vi "Customized NA.vi"() -> ()   [LabVIEW 2021]
panel:
  out "A 2":dbl
  out "A":dbl
  out "Transmission":cluster{"X":dbl, "Y":dbl}[](graph)=[{"X"=1.0, "Y"=0.022832684978800612}, {"X"=1.01, "Y"=-0.03508112044447924}, {"X"=1.02, "Y"=0.011268875649849798}, {"X"=1.03, "Y"=-0.0005874144163142788}, {"X"=1.04, "Y"=-0.013460551415189913}, {"X"=1.05, "Y"=-0.0028755295385605416}, {"X"=1.06, "Y"=-0.01981361181122932}, {"X"=1.07, "Y"=-0.01643174646657092}, {"X"=1.08, "Y"=-0.009902749417672363}, {"X"=1.09, "Y"=0.02696994725538056}, {"X"=1.1, "Y"=0.0013856868529792457}, {"X"=1.11, "Y"=-0.01094619808605209}, {"X"=1.12, "Y"=0.014859773774399874}, {"X"=1.13, "Y"=-0.027897423308499814}, {"X"=1.1400000000000001, "Y"=-0.027737684416107827}, {"X"=1.15, "Y"=0.007918297120363972}, {"X"=1.16, "Y"=-0.018397039322749057}, {"X"=1.17, "Y"=-0.014214660968136495}, {"X"=1.18, "Y"=0.05134840789052823}, {"X"=1.19, "Y"=0.006926672201586222}, {"X"=1.2, "Y"=0.020462736392556753}, {"X"=1.21, "Y"=-0.028066215237332482}, {"X"=1.22, "Y"=-0.02445743439576179}, {"X"=1.23, "Y"=0.03564938650047041}, {"X"=1.24, "Y"=-0.010377576540651738}, {"X"=1.25, "Y"=0.013453196897726083}, {"X"=1.26, "Y"=0.015431438626936772}, {"X"=1.27, "Y"=0.02283777498421219}, {"X"=1.28, "Y"=-0.007799579257767735}, {"X"=1.29, "Y"=0.0234923784994419}, {"X"=1.3, "Y"=0.020565792635922966}, {"X"=1.31, "Y"=0.014042606014675805}, {"X"=1.32, "Y"=-0.00826649286668001}, {"X"=1.33, "Y"=-0.007935280043591663}, {"X"=1.34, "Y"=0.03503153061398124}, {"X"=1.35, "Y"=0.026956957824188083}, {"X"=1.3599999999999999, "Y"=0.029441710251826573}, {"X"=1.37, "Y"=0.03176793153897496}, {"X"=1.38, "Y"=0.02707736760646512}, {"X"=1.3900000000000001, "Y"=0.002384192541336166}, {"X"=1.4, "Y"=-0.0042640262941606175}, {"X"=1.4100000000000001, "Y"=0.05346182081654834}, {"X"=1.42, "Y"=0.03555493439663364}, {"X"=1.43, "Y"=-0.004520863626681091}, {"X"=1.44, "Y"=-0.016774217224386375}, {"X"=1.45, "Y"=-0.005965400673648759}, {"X"=1.46, "Y"=-0.0010894043039113353}, {"X"=1.47, "Y"=-0.00046876709353084185}, {"X"=1.48, "Y"=0.012684810390652803}, {"X"=1.49, "Y"=0.03813067356398994}, {"X"=1.5, "Y"=0.028034897066981875}, {"X"=1.51, "Y"=0.0004972634699936428}, {"X"=1.52, "Y"=-0.00885702548596945}, {"X"=1.53, "Y"=-0.0014397783600446864}, {"X"=1.54, "Y"=0.02559738967135176}, {"X"=1.55, "Y"=0.02940201090770585}, {"X"=1.56, "Y"=-0.00800150373652454}, {"X"=1.57, "Y"=0.006450333329645636}, {"X"=1.58, "Y"=0.004569407290840438}, {"X"=1.5899999999999999, "Y"=-0.000598240579322772}, {"X"=1.6, "Y"=-0.014320673486041196}, {"X"=1.6099999999999999, "Y"=0.0027199883542179957}, {"X"=1.62, "Y"=0.02908043278181352}, {"X"=1.63, "Y"=0.020256081684782996}, {"X"=1.6400000000000001, "Y"=0.014829149563513153}, {"X"=1.65, "Y"=-0.019887629125237172}, {"X"=1.6600000000000001, "Y"=0.04144270630923306}, {"X"=1.67, "Y"=0.055620811367091655}, {"X"=1.6800000000000002, "Y"=-0.05015047761465842}, {"X"=1.69, "Y"=0.016115782004926103}, {"X"=1.7000000000000002, "Y"=0.022219967844359437}, {"X"=1.71, "Y"=-0.019533017885574717}, {"X"=1.72, "Y"=0.002002035002969814}, {"X"=1.73, "Y"=-0.018597470141180916}, {"X"=1.74, "Y"=-0.020507493473050777}, {"X"=1.75, "Y"=0.04497118743572116}, {"X"=1.76, "Y"=-0.03014262884386368}, {"X"=1.77, "Y"=-0.02635719806032388}, {"X"=1.78, "Y"=0.006535826712424916}, {"X"=1.79, "Y"=0.02334340013557594}, {"X"=1.8, "Y"=-0.014584642495372427}, {"X"=1.81, "Y"=0.030318500830231188}, {"X"=1.82, "Y"=0.020334854112019567}, {"X"=1.83, "Y"=0.04329884774917375}, {"X"=1.8399999999999999, "Y"=-0.025542094923208684}, {"X"=1.85, "Y"=0.003997116512462377}, {"X"=1.8599999999999999, "Y"=0.002476500606431811}, {"X"=1.87, "Y"=-0.015934904275146204}, {"X"=1.88, "Y"=0.022274962013573}, {"X"=1.8900000000000001, "Y"=-0.017679939353418044}, {"X"=1.9, "Y"=-0.006070507215851479}, {"X"=1.9100000000000001, "Y"=0.020445304004784615}, {"X"=1.92, "Y"=0.0240972950297685}, {"X"=1.9300000000000002, "Y"=-0.007427137567462293}, {"X"=1.94, "Y"=-0.04383462926305039}, {"X"=1.9500000000000002, "Y"=0.029534523383703232}, {"X"=1.96, "Y"=0.004663156332775081}, {"X"=1.97, "Y"=0.006710309156515723}, {"X"=1.98, "Y"=0.01918446886521864}, {"X"=1.99, "Y"=0.015197749143457322}, {"X"=2.0, "Y"=-0.009373297526692696}, {"X"=2.01, "Y"=-0.020787679571358297}, {"X"=2.02, "Y"=0.010482467499636692}, {"X"=2.0300000000000002, "Y"=-0.005673220895538561}, {"X"=2.04, "Y"=0.043413707084557746}, {"X"=2.05, "Y"=-0.035716121505957696}, {"X"=2.06, "Y"=0.009439154355609746}, {"X"=2.0700000000000003, "Y"=0.024819571500530446}, {"X"=2.08, "Y"=-0.016880198106777607}, {"X"=2.09, "Y"=0.026621278695482094}, {"X"=2.1, "Y"=0.03279616375256214}, {"X"=2.1100000000000003, "Y"=-0.023778293750323753}, {"X"=2.12, "Y"=-0.00758359892975606}, {"X"=2.13, "Y"=0.014366347891758106}, {"X"=2.14, "Y"=0.04279986206549578}, {"X"=2.1500000000000004, "Y"=-0.040135273168241045}, {"X"=2.16, "Y"=0.020430602530422656}, {"X"=2.17, "Y"=-0.01016181476140147}, {"X"=2.1799999999999997, "Y"=0.028271228256628374}, {"X"=2.19, "Y"=0.019003193029244296}, {"X"=2.2, "Y"=0.0008409207192296246}, {"X"=2.21, "Y"=-0.037877245497559386}, {"X"=2.2199999999999998, "Y"=0.0446701137299671}, {"X"=2.23, "Y"=0.06984685412887953}, {"X"=2.24, "Y"=-0.1512091145384057}, {"X"=2.25, "Y"=-0.013116347315476503}, {"X"=2.26, "Y"=0.031777617569120814}, {"X"=2.27, "Y"=0.07416549779761991}, {"X"=2.2800000000000002, "Y"=0.017529876440757167}, {"X"=2.29, "Y"=0.052415560690502835}, {"X"=2.3, "Y"=-0.005680194244753987}, {"X"=2.31, "Y"=-0.018411390213812176}, {"X"=2.3200000000000003, "Y"=-0.026333965630820737}, {"X"=2.33, "Y"=0.06571137750964808}, {"X"=2.34, "Y"=0.0054376541144865115}, {"X"=2.35, "Y"=-0.020271597597055636}, {"X"=2.3600000000000003, "Y"=0.07759004170563122}, {"X"=2.37, "Y"=0.035850286582092966}, {"X"=2.38, "Y"=-0.02336855212013577}, {"X"=2.39, "Y"=0.06239859511241636}, {"X"=2.4000000000000004, "Y"=0.02007528674894494}, {"X"=2.41, "Y"=-0.04739090966025122}, {"X"=2.42, "Y"=-0.08564345665375438}, {"X"=2.4299999999999997, "Y"=-0.013841536597467665}, {"X"=2.44, "Y"=0.0021138229762637088}, {"X"=2.45, "Y"=-0.021017086145964592}, {"X"=2.46, "Y"=-0.020361023579240627}, {"X"=2.4699999999999998, "Y"=0.024491967665518453}, {"X"=2.48, "Y"=0.03218428353928}, {"X"=2.49, "Y"=-0.005050025919170744}, {"X"=2.5, "Y"=0.029742208517415845}, {"X"=2.51, "Y"=0.004789029248200747}, {"X"=2.52, "Y"=-0.13934794980696374}, {"X"=2.5300000000000002, "Y"=-0.03798683524903521}, {"X"=2.54, "Y"=-0.07155314661572079}, {"X"=2.55, "Y"=-0.11201338285103184}, {"X"=2.56, "Y"=0.03928865357098744}, {"X"=2.5700000000000003, "Y"=0.0011758856569439962}, {"X"=2.58, "Y"=-0.0352838332883873}, {"X"=2.59, "Y"=0.016700710042482622}, {"X"=2.6, "Y"=0.0908188603890548}, {"X"=2.6100000000000003, "Y"=0.10223497813700759}, {"X"=2.62, "Y"=-0.04742710381541565}, {"X"=2.63, "Y"=-0.033167276584604784}, {"X"=2.64, "Y"=0.04745249665461672}, {"X"=2.6500000000000004, "Y"=0.025349587473101808}, {"X"=2.66, "Y"=0.017802593659973703}, {"X"=2.67, "Y"=-0.04685585708571281}, {"X"=2.6799999999999997, "Y"=-0.08387314101351168}, {"X"=2.69, "Y"=-0.03234456822103964}, {"X"=2.7, "Y"=0.027006462959568277}, {"X"=2.71, "Y"=0.01950826840478045}, {"X"=2.7199999999999998, "Y"=-0.038306147125277384}, {"X"=2.73, "Y"=-0.04230484199985435}, {"X"=2.74, "Y"=0.10962333038679434}, {"X"=2.75, "Y"=-0.03298581045891181}, {"X"=2.76, "Y"=0.04395085261705363}, {"X"=2.77, "Y"=-0.027711990194185156}, {"X"=2.7800000000000002, "Y"=-0.02334447300823595}, {"X"=2.79, "Y"=-0.043751510055663155}, {"X"=2.8, "Y"=-0.036739162352264695}, {"X"=2.81, "Y"=0.01823108879192129}, {"X"=2.8200000000000003, "Y"=0.04305449107544684}, {"X"=2.83, "Y"=0.027090035845116794}, {"X"=2.84, "Y"=0.048568482476985406}, {"X"=2.85, "Y"=-0.01755577935231485}, {"X"=2.8600000000000003, "Y"=0.07189605462177102}, {"X"=2.87, "Y"=-0.02501098567160028}, {"X"=2.88, "Y"=0.07425676651917856}, {"X"=2.89, "Y"=-0.02027617018909622}, {"X"=2.9000000000000004, "Y"=-0.005896027479349646}, {"X"=2.91, "Y"=0.005746319281931056}, {"X"=2.92, "Y"=-0.03380752673512488}, {"X"=2.9299999999999997, "Y"=0.07941452840444055}, {"X"=2.94, "Y"=0.05078915604914684}, {"X"=2.95, "Y"=0.029856544979316106}, {"X"=2.96, "Y"=-0.03058285055865035}, {"X"=2.9699999999999998, "Y"=-0.04547982494250577}, {"X"=2.98, "Y"=-0.009980119590642253}, {"X"=2.99, "Y"=-0.01818447635229049}, {"X"=3.0, "Y"=0.07945500193940262}, {"X"=3.0100000000000002, "Y"=0.08275405506991075}, {"X"=3.02, "Y"=-0.0034565843835413484}, {"X"=3.0300000000000002, "Y"=0.03628268561148537}, {"X"=3.04, "Y"=0.0850972333719007}, {"X"=3.05, "Y"=0.02617391669515131}, {"X"=3.06, "Y"=0.01305021600187181}, {"X"=3.07, "Y"=-0.06074521733631981}, {"X"=3.08, "Y"=0.04343063137517468}, {"X"=3.09, "Y"=0.02201666314507795}, {"X"=3.1, "Y"=0.0070759706667916115}, {"X"=3.11, "Y"=0.057061180354922796}, {"X"=3.12, "Y"=0.0802501762720645}, {"X"=3.13, "Y"=0.015564742693625188}, {"X"=3.14, "Y"=0.044379698443209686}, {"X"=3.15, "Y"=0.017603055883018654}, {"X"=3.16, "Y"=-0.04071763298347281}, {"X"=3.17, "Y"=0.09096122424136396}, {"X"=3.18, "Y"=0.043580103196136234}, {"X"=3.19, "Y"=-0.09467214131964694}, {"X"=3.2, "Y"=-0.09707522357269399}, {"X"=3.21, "Y"=0.00698445328079356}, {"X"=3.22, "Y"=0.11095283062616748}, {"X"=3.23, "Y"=-0.03926380275146876}, {"X"=3.24, "Y"=-0.03958261403960299}, {"X"=3.25, "Y"=0.1039628104142574}, {"X"=3.2600000000000002, "Y"=-0.0689182435036647}, {"X"=3.27, "Y"=-0.015436043748904043}, {"X"=3.2800000000000002, "Y"=0.08837165232576974}, {"X"=3.29, "Y"=0.058598462680413334}, {"X"=3.3000000000000003, "Y"=0.06659105530606726}, {"X"=3.31, "Y"=-0.08391797405548568}, {"X"=3.32, "Y"=0.0057814891416524935}, {"X"=3.33, "Y"=0.01434772668069612}, {"X"=3.34, "Y"=-0.08232557490042736}, {"X"=3.35, "Y"=0.11618755685481778}, {"X"=3.36, "Y"=-0.0462425691612918}, {"X"=3.37, "Y"=-0.06578870867716782}, {"X"=3.38, "Y"=0.007209182089777069}, {"X"=3.39, "Y"=-0.06691531254049357}, {"X"=3.4, "Y"=-0.060318768636318514}, {"X"=3.41, "Y"=-0.021578326504440092}, {"X"=3.42, "Y"=0.0852333266694384}, {"X"=3.43, "Y"=0.02308479726231716}, {"X"=3.44, "Y"=0.0075950328899135515}, {"X"=3.45, "Y"=-0.03412596564957042}, {"X"=3.46, "Y"=0.003918703423516029}, {"X"=3.47, "Y"=-0.007266144246662869}, {"X"=3.48, "Y"=-0.045965202132127084}, {"X"=3.49, "Y"=0.01126270144189599}, {"X"=3.5, "Y"=-0.024950149108312617}, {"X"=3.5100000000000002, "Y"=-0.004967585360949168}, {"X"=3.52, "Y"=-0.03350851808015104}, {"X"=3.5300000000000002, "Y"=0.021208062347619946}, {"X"=3.54, "Y"=0.006769935405607826}, {"X"=3.5500000000000003, "Y"=0.0006168657836808115}, {"X"=3.56, "Y"=-0.015220609363573584}, {"X"=3.57, "Y"=0.05611405954327623}, {"X"=3.58, "Y"=-0.0017864784435978735}, {"X"=3.59, "Y"=0.06640041965890024}, {"X"=3.6, "Y"=-0.062001646665789605}, {"X"=3.61, "Y"=0.0407690793988466}, {"X"=3.62, "Y"=-0.0042725893684103355}, {"X"=3.63, "Y"=-0.0025174649352865566}, {"X"=3.64, "Y"=0.05581022456125648}, {"X"=3.65, "Y"=0.011370620056615965}, {"X"=3.66, "Y"=-0.04200147567669391}, {"X"=3.67, "Y"=0.010578324850903396}, {"X"=3.68, "Y"=0.040859849306499045}, {"X"=3.69, "Y"=-0.005526197538349407}, {"X"=3.7, "Y"=-0.01617682054741165}, {"X"=3.71, "Y"=0.07269032354718705}, {"X"=3.72, "Y"=-0.05776232666288099}, {"X"=3.73, "Y"=-0.004728688639122597}, {"X"=3.74, "Y"=0.002597162426423107}, {"X"=3.75, "Y"=-0.026489101251556235}, {"X"=3.7600000000000002, "Y"=0.030955691217215288}, {"X"=3.77, "Y"=0.023385540849718688}, {"X"=3.7800000000000002, "Y"=0.027553894482035306}, {"X"=3.79, "Y"=-0.09409366427804487}, {"X"=3.8000000000000003, "Y"=-0.06792668801725968}, {"X"=3.81, "Y"=-0.03865762834406878}, {"X"=3.82, "Y"=-0.01811856693051703}, {"X"=3.83, "Y"=0.003927659612420333}, {"X"=3.84, "Y"=-0.010097980566907357}, {"X"=3.85, "Y"=-0.023977943851357462}, {"X"=3.86, "Y"=0.06520359414384269}, {"X"=3.87, "Y"=-0.03661154466253325}, {"X"=3.88, "Y"=0.03527993069682999}, {"X"=3.89, "Y"=-0.011199826840143904}, {"X"=3.9, "Y"=0.050607938195409465}, {"X"=3.91, "Y"=-0.021860793111017074}, {"X"=3.92, "Y"=-0.01721744336974712}, {"X"=3.93, "Y"=-0.013840547783161017}, {"X"=3.94, "Y"=0.0691868524990469}, {"X"=3.95, "Y"=-0.06902153851771764}, {"X"=3.96, "Y"=-0.07989983105634205}, {"X"=3.97, "Y"=0.058072220827240825}, {"X"=3.98, "Y"=-0.0449358670835874}, {"X"=3.99, "Y"=-0.05881172212666866}, {"X"=4.0, "Y"=0.007012843202961465}, {"X"=4.01, "Y"=-0.01976886944251683}, {"X"=4.02, "Y"=0.12155819256128322}, {"X"=4.03, "Y"=-0.0250454630119111}, {"X"=4.04, "Y"=-0.027790584747937403}, {"X"=4.050000000000001, "Y"=0.045072481686222965}, {"X"=4.0600000000000005, "Y"=-0.01660556663787395}, {"X"=4.07, "Y"=0.004334820947334434}, {"X"=4.08, "Y"=0.0499033828292426}, {"X"=4.09, "Y"=-0.033615562408676566}, {"X"=4.1, "Y"=0.08021788774986288}, {"X"=4.109999999999999, "Y"=0.038023100278270945}, {"X"=4.12, "Y"=0.03143250107624138}, {"X"=4.13, "Y"=0.044455122360404976}, {"X"=4.140000000000001, "Y"=-0.010891177933356803}, {"X"=4.15, "Y"=-0.017043647532097878}, {"X"=4.16, "Y"=0.0004046636993076181}, {"X"=4.17, "Y"=-0.05218873623384405}, {"X"=4.18, "Y"=0.04061672976652943}, {"X"=4.1899999999999995, "Y"=0.01650703203746078}, {"X"=4.2, "Y"=0.02050704058903572}, {"X"=4.21, "Y"=0.008880269535492638}, {"X"=4.220000000000001, "Y"=-0.04762701769693031}, {"X"=4.23, "Y"=-0.03040919031812101}, {"X"=4.24, "Y"=0.055623259921242334}, {"X"=4.25, "Y"=-0.0869295634531754}, {"X"=4.26, "Y"=0.008701771845440135}, {"X"=4.27, "Y"=0.10651722648351944}, {"X"=4.28, "Y"=-0.09324931771576475}, {"X"=4.29, "Y"=-0.04867438076276051}, {"X"=4.300000000000001, "Y"=0.05172230475947215}, {"X"=4.3100000000000005, "Y"=-0.03132172955212597}, {"X"=4.32, "Y"=0.0005489734925474995}, {"X"=4.33, "Y"=0.05785080404470754}, {"X"=4.34, "Y"=0.0774941869504657}, {"X"=4.35, "Y"=-0.07565540752815414}, {"X"=4.359999999999999, "Y"=0.006617263677769838}, {"X"=4.37, "Y"=-0.020981681602773278}, {"X"=4.38, "Y"=0.035442905708659114}, {"X"=4.390000000000001, "Y"=0.004263421468070699}, {"X"=4.4, "Y"=-0.06029702743738625}, {"X"=4.41, "Y"=0.058822033155191}, {"X"=4.42, "Y"=0.021382590561579394}, {"X"=4.43, "Y"=0.09092874009495779}, {"X"=4.4399999999999995, "Y"=0.06753347213354402}, {"X"=4.45, "Y"=0.03013462443441948}, {"X"=4.46, "Y"=0.03745075402786496}, {"X"=4.470000000000001, "Y"=-0.04660006949267839}, {"X"=4.48, "Y"=0.005508048389048581}, {"X"=4.49, "Y"=0.043115471876064876}, {"X"=4.5, "Y"=-0.0871176462869269}, {"X"=4.51, "Y"=0.07586308305437081}, {"X"=4.52, "Y"=0.022715616729637452}, {"X"=4.53, "Y"=-0.01727572277141465}, {"X"=4.54, "Y"=-0.03794965009767242}, {"X"=4.550000000000001, "Y"=0.010055728758651933}, {"X"=4.5600000000000005, "Y"=0.03202629537262217}, {"X"=4.57, "Y"=-0.07704800319642835}, {"X"=4.58, "Y"=0.0927616651714244}, {"X"=4.59, "Y"=0.09892908927815028}, {"X"=4.6, "Y"=-0.05991396658646459}, {"X"=4.609999999999999, "Y"=0.08111216389687827}, {"X"=4.62, "Y"=0.012048658974672041}, {"X"=4.63, "Y"=-0.04193418179011241}, {"X"=4.640000000000001, "Y"=-0.04397480041967557}, {"X"=4.65, "Y"=0.0680685572436193}, {"X"=4.66, "Y"=-0.06799288425132947}, {"X"=4.67, "Y"=0.02560055056292842}, {"X"=4.68, "Y"=-0.04321943957399119}, {"X"=4.6899999999999995, "Y"=-0.0614936122954018}, {"X"=4.7, "Y"=0.018843901456124055}, {"X"=4.71, "Y"=0.06008977829647717}, {"X"=4.720000000000001, "Y"=-0.11646958930016804}, {"X"=4.73, "Y"=0.0856022095141052}, {"X"=4.74, "Y"=-0.06638889684464488}, {"X"=4.75, "Y"=0.03596862802600055}, {"X"=4.76, "Y"=-0.021352879962272562}, {"X"=4.77, "Y"=0.06888410676873159}, {"X"=4.78, "Y"=0.0898034986792025}, {"X"=4.79, "Y"=0.011212490772019426}, {"X"=4.800000000000001, "Y"=-0.06778172263811245}, {"X"=4.8100000000000005, "Y"=-0.0033927133747117355}, {"X"=4.82, "Y"=-0.04228825125694992}, {"X"=4.83, "Y"=0.051201590327728974}, {"X"=4.84, "Y"=0.006469950932159545}, {"X"=4.85, "Y"=-0.004096290348928243}, {"X"=4.859999999999999, "Y"=-0.040305885103016706}, {"X"=4.87, "Y"=-0.002746560238113844}, {"X"=4.88, "Y"=0.07497410641651443}, {"X"=4.890000000000001, "Y"=-0.0610580809789402}, {"X"=4.9, "Y"=-0.0804416331724484}, {"X"=4.91, "Y"=0.10151325466932744}, {"X"=4.92, "Y"=-0.0676234696057146}, {"X"=4.93, "Y"=-0.08309292898981475}, {"X"=4.9399999999999995, "Y"=-0.07214345078025752}, {"X"=4.95, "Y"=-0.023729642314904393}, {"X"=4.96, "Y"=0.06344203528926698}, {"X"=4.970000000000001, "Y"=-0.05805387668942516}, {"X"=4.98, "Y"=0.004000411346397273}, {"X"=4.99, "Y"=-0.018205862104963628}, {"X"=5.0, "Y"=-0.02825625557825697}, {"X"=5.01, "Y"=0.06687188014055709}, {"X"=5.0200000000000005, "Y"=-0.07402043889823232}, {"X"=5.03, "Y"=-0.0017328200543095212}, {"X"=5.04, "Y"=0.004094617484746082}, {"X"=5.05, "Y"=0.04056662094713038}, {"X"=5.0600000000000005, "Y"=0.07031583013095852}, {"X"=5.07, "Y"=-0.08400005811035077}, {"X"=5.08, "Y"=0.004835897661026842}, {"X"=5.09, "Y"=-0.0068396947676980496}, {"X"=5.1, "Y"=-0.03895606869887244}, {"X"=5.11, "Y"=-0.0660495051717288}, {"X"=5.12, "Y"=0.01788466628936112}, {"X"=5.13, "Y"=-0.01011945117972266}, {"X"=5.14, "Y"=0.07368085432335891}, {"X"=5.15, "Y"=0.06516614983388168}, {"X"=5.16, "Y"=0.05233099658608864}, {"X"=5.17, "Y"=0.02019717251794414}, {"X"=5.18, "Y"=0.006497754963668157}, {"X"=5.19, "Y"=-0.003948603096509178}, {"X"=5.2, "Y"=6.661568501261176e-05}, {"X"=5.21, "Y"=-0.01279925443863473}, {"X"=5.22, "Y"=-0.008656479795343144}, {"X"=5.23, "Y"=0.07785688499876349}, {"X"=5.24, "Y"=-0.08473584480229832}, {"X"=5.25, "Y"=0.01476928463721575}, {"X"=5.26, "Y"=-0.022658354624478412}, {"X"=5.2700000000000005, "Y"=0.02327650125462502}, {"X"=5.28, "Y"=0.062584133132754}, {"X"=5.29, "Y"=0.03794044335539621}, {"X"=5.3, "Y"=-0.016801229929570484}, {"X"=5.3100000000000005, "Y"=-0.015286291444591486}, {"X"=5.32, "Y"=0.008384772747949692}, {"X"=5.33, "Y"=-0.03301969193302869}, {"X"=5.34, "Y"=-0.02266876409030525}, {"X"=5.3500000000000005, "Y"=-0.00576491681118074}, {"X"=5.36, "Y"=-0.05552363297354124}, {"X"=5.37, "Y"=-0.013006367872802849}, {"X"=5.38, "Y"=0.05373119511882067}, {"X"=5.39, "Y"=-0.050001439273800706}, {"X"=5.4, "Y"=0.08567964785833415}, {"X"=5.41, "Y"=0.013840917058350341}, {"X"=5.42, "Y"=-0.02718554399906313}, {"X"=5.43, "Y"=0.06063616944576644}, {"X"=5.44, "Y"=0.08130753009647768}, {"X"=5.45, "Y"=0.005634360665437893}, {"X"=5.46, "Y"=-0.026023479110728335}, {"X"=5.47, "Y"=-0.06883190413201781}, {"X"=5.48, "Y"=0.02330407465252426}, {"X"=5.49, "Y"=-0.011808862231552397}, {"X"=5.5, "Y"=-0.02791573176101704}, {"X"=5.51, "Y"=0.024218182285824282}, {"X"=5.5200000000000005, "Y"=-0.07318363884626461}, {"X"=5.53, "Y"=0.014776116088776218}, {"X"=5.54, "Y"=0.05307232307193971}, {"X"=5.55, "Y"=0.047698246364990336}, {"X"=5.5600000000000005, "Y"=-0.10501889985819901}, {"X"=5.57, "Y"=-0.014264400829335385}, {"X"=5.58, "Y"=0.05638892090314287}, {"X"=5.59, "Y"=-0.05727734536015227}, {"X"=5.6000000000000005, "Y"=-0.030205628406936767}, {"X"=5.61, "Y"=-0.012312298439080736}, {"X"=5.62, "Y"=-0.05648910235162506}, {"X"=5.63, "Y"=0.019853004960957717}, {"X"=5.64, "Y"=-0.013361219454529496}, {"X"=5.65, "Y"=-0.024642502677854686}, {"X"=5.66, "Y"=-0.0036450627420398767}, {"X"=5.67, "Y"=-0.008268604296393551}, {"X"=5.68, "Y"=0.02327261388447934}, {"X"=5.69, "Y"=-0.018620728308615886}, {"X"=5.7, "Y"=-0.08158408138084744}, {"X"=5.71, "Y"=0.023297617121373272}, {"X"=5.72, "Y"=0.07595893524808649}, {"X"=5.73, "Y"=0.07320145431186481}, {"X"=5.74, "Y"=0.017981129889461104}, {"X"=5.75, "Y"=-0.0040682283071078705}, {"X"=5.76, "Y"=-0.0010420723545586708}, {"X"=5.7700000000000005, "Y"=-0.024547762025628618}, {"X"=5.78, "Y"=-0.012665919576779268}, {"X"=5.79, "Y"=-0.005197627918570575}, {"X"=5.8, "Y"=-0.06611686856976666}, {"X"=5.8100000000000005, "Y"=0.022296312910474063}, {"X"=5.82, "Y"=-0.04294412319333043}, {"X"=5.83, "Y"=0.022626652659306374}, {"X"=5.84, "Y"=-0.029854165783535818}, {"X"=5.8500000000000005, "Y"=-0.06070624733299346}, {"X"=5.86, "Y"=0.01956199148189994}, {"X"=5.87, "Y"=-0.012973060237718817}, {"X"=5.88, "Y"=-0.003070477388174685}, {"X"=5.89, "Y"=0.11267036770815719}, {"X"=5.9, "Y"=-0.052035006895199444}, {"X"=5.91, "Y"=-0.002651315993240094}, {"X"=5.92, "Y"=-0.00834646331838685}, {"X"=5.93, "Y"=-0.022085885029240512}, {"X"=5.94, "Y"=0.101802055065484}, {"X"=5.95, "Y"=0.0010665126497984149}, {"X"=5.96, "Y"=-0.009677063350274509}, {"X"=5.97, "Y"=-0.022015735571015674}, {"X"=5.98, "Y"=-0.03138576962189697}, {"X"=5.99, "Y"=-0.01987837444026668}, {"X"=6.0, "Y"=-0.04907590695717144}, {"X"=6.01, "Y"=-0.0077242036923909135}, {"X"=6.0200000000000005, "Y"=-0.05782383063626509}, {"X"=6.03, "Y"=0.02704462328516077}, {"X"=6.04, "Y"=0.09307068498329031}, {"X"=6.05, "Y"=-0.0488201120234237}, {"X"=6.0600000000000005, "Y"=0.0636734230861321}, {"X"=6.07, "Y"=0.0012186305735722165}, {"X"=6.08, "Y"=-0.036398306376224196}, {"X"=6.09, "Y"=0.06597376581416425}, {"X"=6.1000000000000005, "Y"=-0.06972096234108914}, {"X"=6.11, "Y"=0.033811098550895625}, {"X"=6.12, "Y"=-0.014381684403489626}, {"X"=6.13, "Y"=-0.03719238572359069}, {"X"=6.14, "Y"=0.029041839234955378}, {"X"=6.15, "Y"=0.017315147772606863}, {"X"=6.16, "Y"=0.07123969578901798}, {"X"=6.17, "Y"=-0.06650408681575551}, {"X"=6.18, "Y"=-0.0849044750000516}, {"X"=6.19, "Y"=0.0021684158556381883}, {"X"=6.2, "Y"=0.10249108922219508}, {"X"=6.21, "Y"=-0.05627004052995942}, {"X"=6.22, "Y"=0.028328814356917136}, {"X"=6.23, "Y"=-0.015705872082460534}, {"X"=6.24, "Y"=-0.011995009024246791}, {"X"=6.25, "Y"=-0.03467250107688492}, {"X"=6.26, "Y"=-0.01861613676447849}, {"X"=6.2700000000000005, "Y"=-0.05448718465813741}, {"X"=6.28, "Y"=0.026397454317599767}, {"X"=6.29, "Y"=0.006047020172822425}, {"X"=6.3, "Y"=-0.02063257330634548}, {"X"=6.3100000000000005, "Y"=0.04820225957752912}, {"X"=6.32, "Y"=0.0031330571855591118}, {"X"=6.33, "Y"=-0.0751085738089421}, {"X"=6.34, "Y"=0.044869273139189716}, {"X"=6.3500000000000005, "Y"=-0.10399176378801499}, {"X"=6.36, "Y"=0.07796981446277082}, {"X"=6.37, "Y"=-0.09860711006539849}, {"X"=6.38, "Y"=0.0031854750277705993}, {"X"=6.39, "Y"=0.007679172017556302}, {"X"=6.4, "Y"=0.025637240545327553}, {"X"=6.41, "Y"=-0.054181986021784485}, {"X"=6.42, "Y"=0.0527404808334727}, {"X"=6.43, "Y"=0.02313301859817469}, {"X"=6.44, "Y"=0.026221241277444}, {"X"=6.45, "Y"=-0.02964563954650836}, {"X"=6.46, "Y"=0.031768954773586926}, {"X"=6.47, "Y"=-0.01573579654135559}, {"X"=6.48, "Y"=-0.040580328220727886}, {"X"=6.49, "Y"=-0.02662585632207066}, {"X"=6.5, "Y"=-0.09071657947456498}, {"X"=6.51, "Y"=0.008280037158494792}, {"X"=6.5200000000000005, "Y"=0.11283699459805265}, {"X"=6.53, "Y"=-0.07868477427490554}, {"X"=6.54, "Y"=-0.0262246362037586}, {"X"=6.55, "Y"=-0.06964792688719483}, {"X"=6.5600000000000005, "Y"=0.035030527879914015}, {"X"=6.57, "Y"=0.0606362841420183}, {"X"=6.58, "Y"=0.0006396530299344917}, {"X"=6.59, "Y"=-0.052298831531626545}, {"X"=6.6000000000000005, "Y"=0.02485867814693695}, {"X"=6.61, "Y"=-0.0014104222272999292}, {"X"=6.62, "Y"=-0.02253256190494117}, {"X"=6.63, "Y"=-0.014940416142262953}, {"X"=6.64, "Y"=0.05528729358180156}, {"X"=6.65, "Y"=-0.0018451076868453446}, {"X"=6.66, "Y"=-0.03183482858233051}, {"X"=6.67, "Y"=-0.0733775395365832}, {"X"=6.68, "Y"=-0.07553121895390386}, {"X"=6.69, "Y"=-0.022418086123786866}, {"X"=6.7, "Y"=0.0395888641713284}, {"X"=6.71, "Y"=0.018122486711339123}, {"X"=6.72, "Y"=0.015738618550992678}, {"X"=6.73, "Y"=0.04716569134894259}, {"X"=6.74, "Y"=0.008485389867849058}, {"X"=6.75, "Y"=-0.0008077875922679607}, {"X"=6.76, "Y"=-0.032377926874882904}, {"X"=6.7700000000000005, "Y"=0.03393815781202512}, {"X"=6.78, "Y"=0.006267170732572651}, {"X"=6.79, "Y"=-0.007785689846387309}, {"X"=6.8, "Y"=-0.02878104897484103}, {"X"=6.8100000000000005, "Y"=0.06825915171098933}, {"X"=6.82, "Y"=-0.09185848137386607}, {"X"=6.83, "Y"=-0.07251419366033288}, {"X"=6.84, "Y"=0.005698805677795994}, {"X"=6.8500000000000005, "Y"=-0.04703857507298587}, {"X"=6.86, "Y"=-0.019491653575998406}, {"X"=6.87, "Y"=-0.0040874031203206925}, {"X"=6.88, "Y"=-0.07990260505532659}, {"X"=6.89, "Y"=0.015685900822169682}, {"X"=6.9, "Y"=0.03955455575520666}, {"X"=6.91, "Y"=-0.012866684049411867}, {"X"=6.92, "Y"=-0.018480191376442794}, {"X"=6.93, "Y"=-0.00796299797686319}, {"X"=6.94, "Y"=0.029148320301354207}, {"X"=6.95, "Y"=0.03323884851645199}, {"X"=6.96, "Y"=-0.01666489185418468}, {"X"=6.97, "Y"=-0.032860701352025984}, {"X"=6.98, "Y"=0.06956150407066317}, {"X"=6.99, "Y"=-0.08615764337072454}, {"X"=7.0, "Y"=-0.025492306255667035}, {"X"=7.01, "Y"=0.03545609363378677}, {"X"=7.0200000000000005, "Y"=0.04386140016404986}, {"X"=7.03, "Y"=-0.006628044442995146}, {"X"=7.04, "Y"=0.005739242814838712}, {"X"=7.05, "Y"=-0.017825405935535825}, {"X"=7.0600000000000005, "Y"=-0.050609198327390664}, {"X"=7.07, "Y"=0.02501886036138073}, {"X"=7.08, "Y"=0.0003467243515429132}, {"X"=7.09, "Y"=-0.03157639522157096}, {"X"=7.1000000000000005, "Y"=-0.02849820502133508}, {"X"=7.11, "Y"=0.013270008751749104}, {"X"=7.12, "Y"=-0.015437688381877137}, {"X"=7.13, "Y"=0.03772687734633346}, {"X"=7.140000000000001, "Y"=-0.07144710000749377}, {"X"=7.15, "Y"=-0.048141155629827306}, {"X"=7.16, "Y"=-0.027118297282748557}, {"X"=7.17, "Y"=-0.04420239489899797}, {"X"=7.18, "Y"=0.007697768806045778}, {"X"=7.19, "Y"=-0.011890603856907475}, {"X"=7.2, "Y"=-0.026849987295301067}, {"X"=7.21, "Y"=0.03211334233562174}, {"X"=7.22, "Y"=0.04059918351565901}, {"X"=7.23, "Y"=0.013459884950961025}, {"X"=7.24, "Y"=-0.021369795035309905}, {"X"=7.25, "Y"=-0.021545164361347513}, {"X"=7.26, "Y"=-0.03632116899760873}, {"X"=7.2700000000000005, "Y"=-0.03233424475057812}, {"X"=7.28, "Y"=0.02727282976611005}, {"X"=7.29, "Y"=-0.005760338430239383}, {"X"=7.3, "Y"=0.07053393564875293}, {"X"=7.3100000000000005, "Y"=0.06534257024727654}, {"X"=7.32, "Y"=-0.04744976010407371}, {"X"=7.33, "Y"=0.03478918855596757}, {"X"=7.34, "Y"=0.007466189032604985}, {"X"=7.3500000000000005, "Y"=-0.015353452863796904}, {"X"=7.36, "Y"=-0.02032624048054464}, {"X"=7.37, "Y"=-0.03459465756313689}, {"X"=7.38, "Y"=0.006731100383444488}, {"X"=7.390000000000001, "Y"=0.02723783798457087}, {"X"=7.4, "Y"=0.0311717319145719}, {"X"=7.41, "Y"=0.017412408428444194}, {"X"=7.42, "Y"=-0.000598127849227487}, {"X"=7.43, "Y"=-0.02333005933454644}, {"X"=7.44, "Y"=0.05791851945272888}, {"X"=7.45, "Y"=0.06277219060154157}, {"X"=7.46, "Y"=-0.06053876359352548}, {"X"=7.47, "Y"=-0.008085140611526905}, {"X"=7.48, "Y"=-0.016086808817817978}, {"X"=7.49, "Y"=-0.05268465937705026}, {"X"=7.5, "Y"=0.024604862170655446}, {"X"=7.51, "Y"=-0.0009583081405395998}, {"X"=7.5200000000000005, "Y"=-0.023407761945125415}, {"X"=7.53, "Y"=0.04168242776930939}, {"X"=7.54, "Y"=0.005273366465996269}, {"X"=7.55, "Y"=-0.033647233270786066}, {"X"=7.5600000000000005, "Y"=0.049223179029174724}, {"X"=7.57, "Y"=-0.0009277275568955718}, {"X"=7.58, "Y"=-0.014411339272251175}, {"X"=7.59, "Y"=-0.022242772588406755}, {"X"=7.6000000000000005, "Y"=0.023720029368191432}, {"X"=7.61, "Y"=-0.029086488466908332}, {"X"=7.62, "Y"=0.08052666302272937}, {"X"=7.63, "Y"=0.034573439728877615}, {"X"=7.640000000000001, "Y"=-0.052033654506892714}, {"X"=7.65, "Y"=-0.042549762405956794}, {"X"=7.66, "Y"=0.034488747819776}, {"X"=7.67, "Y"=-0.020022198818326092}, {"X"=7.68, "Y"=0.033103564465580375}, {"X"=7.69, "Y"=0.037216338797015594}, {"X"=7.7, "Y"=0.05004949590523347}, {"X"=7.71, "Y"=-0.05459337767384034}, {"X"=7.72, "Y"=0.04820206162331538}, {"X"=7.73, "Y"=-0.034348376516023855}, {"X"=7.74, "Y"=0.07166880790785955}, {"X"=7.75, "Y"=0.036794991031259695}, {"X"=7.76, "Y"=-0.11170575499748828}, {"X"=7.7700000000000005, "Y"=0.003994338384303684}, {"X"=7.78, "Y"=0.07608298688340125}, {"X"=7.79, "Y"=-0.09647127988920767}, {"X"=7.8, "Y"=-0.01285877848063188}, {"X"=7.8100000000000005, "Y"=-0.010716777795334503}, {"X"=7.82, "Y"=0.00849602919438492}, {"X"=7.83, "Y"=-0.020997632753000272}, {"X"=7.84, "Y"=-0.011963032508259506}, {"X"=7.8500000000000005, "Y"=0.05593772067162062}, {"X"=7.86, "Y"=0.03488355555242282}, {"X"=7.87, "Y"=0.043570054426161894}, {"X"=7.88, "Y"=0.0001581509246212246}, {"X"=7.890000000000001, "Y"=0.03274393697827751}, {"X"=7.9, "Y"=0.051857832013972135}, {"X"=7.91, "Y"=-0.0200334790225314}, {"X"=7.92, "Y"=-0.026417155742713014}, {"X"=7.93, "Y"=0.04097749798946947}, {"X"=7.94, "Y"=0.05048551507473313}, {"X"=7.95, "Y"=0.002175982961887432}, {"X"=7.96, "Y"=-0.043616522238223696}, {"X"=7.97, "Y"=0.0120209046091567}, {"X"=7.98, "Y"=-0.007545041887490105}, {"X"=7.99, "Y"=0.029001749097890207}, {"X"=8.0, "Y"=0.023834845820197053}, {"X"=8.01, "Y"=-6.653294777303923e-05}, {"X"=8.02, "Y"=0.03858155501505267}, {"X"=8.030000000000001, "Y"=-0.03591710992125389}, {"X"=8.04, "Y"=-0.01555466545908814}, {"X"=8.05, "Y"=-0.0008109039054409939}, {"X"=8.06, "Y"=-0.07031628376768641}, {"X"=8.07, "Y"=-0.04393648979080937}, {"X"=8.08, "Y"=-0.03976926450381605}, {"X"=8.09, "Y"=-0.0010898211870169127}, {"X"=8.100000000000001, "Y"=0.10005213031132422}, {"X"=8.11, "Y"=0.04377683479760592}, {"X"=8.120000000000001, "Y"=-0.049993084837559106}, {"X"=8.129999999999999, "Y"=0.052602326752118754}, {"X"=8.14, "Y"=-0.020674503283926515}, {"X"=8.15, "Y"=0.019034536206921297}, {"X"=8.16, "Y"=0.01217970107896198}, {"X"=8.17, "Y"=-0.03250876329110408}, {"X"=8.18, "Y"=0.01604275206698287}, {"X"=8.190000000000001, "Y"=0.0938965949651398}, {"X"=8.2, "Y"=0.07699588978072963}, {"X"=8.21, "Y"=-0.05592433234703832}, {"X"=8.219999999999999, "Y"=0.03348057408026266}, {"X"=8.23, "Y"=-0.03435517783144619}, {"X"=8.24, "Y"=0.03814644208924757}, {"X"=8.25, "Y"=0.04154225444586611}, {"X"=8.26, "Y"=0.021386639294740432}, {"X"=8.27, "Y"=-0.012141651051893259}, {"X"=8.280000000000001, "Y"=0.08914138856047166}, {"X"=8.29, "Y"=0.024034343331510718}, {"X"=8.3, "Y"=0.0009399379893656703}, {"X"=8.31, "Y"=0.013912811294547951}, {"X"=8.32, "Y"=0.013009435098767909}, {"X"=8.33, "Y"=0.07321237561496367}, {"X"=8.34, "Y"=-0.0635971491463271}, {"X"=8.350000000000001, "Y"=0.03968624172953179}, {"X"=8.36, "Y"=0.015144086933604741}, {"X"=8.370000000000001, "Y"=0.008747479771298493}, {"X"=8.379999999999999, "Y"=-0.015257453521027387}, {"X"=8.39, "Y"=0.06845175582264554}, {"X"=8.4, "Y"=0.0045535585720400855}, {"X"=8.41, "Y"=-0.029565011859417345}, {"X"=8.42, "Y"=-0.04697776292414026}, {"X"=8.43, "Y"=0.0637449293938879}, {"X"=8.440000000000001, "Y"=0.014089856968485111}, {"X"=8.45, "Y"=0.07717386706606216}, {"X"=8.46, "Y"=-0.006528519371987542}, {"X"=8.469999999999999, "Y"=0.08933454501311104}, {"X"=8.48, "Y"=0.01919044502508877}, {"X"=8.49, "Y"=0.016318203861878426}, {"X"=8.5, "Y"=0.033070908266956855}, {"X"=8.51, "Y"=-0.04780355801198371}, {"X"=8.52, "Y"=0.04560526471349874}, {"X"=8.530000000000001, "Y"=0.004420948870403642}, {"X"=8.54, "Y"=-0.03186841210070628}, {"X"=8.55, "Y"=0.026508683217246393}, {"X"=8.56, "Y"=-0.03199375683776707}, {"X"=8.57, "Y"=0.038494133195179095}, {"X"=8.58, "Y"=0.003942035338913783}, {"X"=8.59, "Y"=0.0022473111245716526}, {"X"=8.600000000000001, "Y"=0.023489168085522833}, {"X"=8.61, "Y"=-0.06555164050340138}, {"X"=8.620000000000001, "Y"=0.06925085721957587}, {"X"=8.629999999999999, "Y"=0.02734496216689024}, {"X"=8.64, "Y"=-0.012550946203266081}, {"X"=8.65, "Y"=-0.011577118316600523}, {"X"=8.66, "Y"=-0.019456458502877114}, {"X"=8.67, "Y"=-0.02834767357124993}, {"X"=8.68, "Y"=-0.032585223262190224}, {"X"=8.690000000000001, "Y"=-0.018595463760622488}, {"X"=8.7, "Y"=0.026930395580891386}, {"X"=8.71, "Y"=0.020936363416889092}, {"X"=8.719999999999999, "Y"=0.04164737537526532}, {"X"=8.73, "Y"=0.002772616009061677}, {"X"=8.74, "Y"=-0.0019243624623548707}, {"X"=8.75, "Y"=0.03646037621554924}, {"X"=8.76, "Y"=-0.0207684002399707}, {"X"=8.77, "Y"=-0.02749520856944925}, {"X"=8.780000000000001, "Y"=0.03139604851828949}, {"X"=8.79, "Y"=0.008088662444068886}, {"X"=8.8, "Y"=-0.03662113518667255}, {"X"=8.81, "Y"=0.04802929094042516}, {"X"=8.82, "Y"=0.024313341535128204}, {"X"=8.83, "Y"=0.030336209832850323}, {"X"=8.84, "Y"=-0.028628833525473494}, {"X"=8.850000000000001, "Y"=0.026735154695654056}, {"X"=8.86, "Y"=-0.03058567384472056}, {"X"=8.870000000000001, "Y"=0.005904402502170359}, {"X"=8.879999999999999, "Y"=0.034505429266217046}, {"X"=8.89, "Y"=0.02511242213060981}, {"X"=8.9, "Y"=-0.026140647939282953}, {"X"=8.91, "Y"=0.03156621239419539}, {"X"=8.92, "Y"=-0.03817143171397274}, {"X"=8.93, "Y"=0.007722748841174593}, {"X"=8.940000000000001, "Y"=-0.04149882667701539}, {"X"=8.95, "Y"=0.03434604627478957}, {"X"=8.96, "Y"=-0.01995470474038627}, {"X"=8.969999999999999, "Y"=-0.042599893483545134}, {"X"=8.98, "Y"=0.02124063770440933}, {"X"=8.99, "Y"=-0.014195972378335428}, {"X"=9.0, "Y"=-0.03502850355778302}, {"X"=9.01, "Y"=0.028767394954683497}, {"X"=9.02, "Y"=-0.02233331991112293}, {"X"=9.03, "Y"=0.028014649822821893}, {"X"=9.040000000000001, "Y"=0.010860196898595893}, {"X"=9.05, "Y"=0.015358949334635543}, {"X"=9.06, "Y"=-0.01801823615278216}, {"X"=9.07, "Y"=-0.04728970482264712}, {"X"=9.08, "Y"=-0.02842056146128643}, {"X"=9.09, "Y"=-0.019637474205094627}, {"X"=9.1, "Y"=-0.0238093764433529}, {"X"=9.11, "Y"=-0.03759151717987686}, {"X"=9.120000000000001, "Y"=0.02585999678042305}, {"X"=9.13, "Y"=-0.03167676070323856}, {"X"=9.14, "Y"=0.02531796593149381}, {"X"=9.15, "Y"=-0.013351865030363678}, {"X"=9.16, "Y"=-0.0009755960931268694}, {"X"=9.17, "Y"=0.04191001354479477}, {"X"=9.18, "Y"=0.005365755138728228}, {"X"=9.19, "Y"=0.026556693531331162}, {"X"=9.2, "Y"=-0.0025404385785716306}, {"X"=9.21, "Y"=-0.027859606829445757}, {"X"=9.22, "Y"=-0.03033579938783129}, {"X"=9.23, "Y"=0.024809914967852082}, {"X"=9.24, "Y"=0.029062062446244645}, {"X"=9.25, "Y"=-0.023985102982247295}, {"X"=9.26, "Y"=-0.03246754209710874}, {"X"=9.27, "Y"=0.0445603214810721}, {"X"=9.28, "Y"=-0.0017856249612823462}, {"X"=9.290000000000001, "Y"=-0.011926674086726772}, {"X"=9.3, "Y"=-0.004272808677014768}, {"X"=9.31, "Y"=-0.015914879661600535}, {"X"=9.32, "Y"=0.0437532955028503}, {"X"=9.33, "Y"=-0.03231280346494594}, {"X"=9.34, "Y"=0.01625302344138455}, {"X"=9.35, "Y"=0.01589336512895472}, {"X"=9.36, "Y"=-0.03963327006185689}, {"X"=9.370000000000001, "Y"=-0.02040792206006905}, {"X"=9.38, "Y"=0.01737657832792597}, {"X"=9.39, "Y"=-0.013904532449061622}, {"X"=9.4, "Y"=-0.03434975071259634}, {"X"=9.41, "Y"=0.019228897683036407}, {"X"=9.42, "Y"=-0.0380988400061366}, {"X"=9.43, "Y"=-0.0005981376375349483}, {"X"=9.44, "Y"=-0.05197507519621772}, {"X"=9.45, "Y"=0.011613299031687853}, {"X"=9.46, "Y"=0.0029584671655475884}, {"X"=9.47, "Y"=0.027537954980181634}, {"X"=9.48, "Y"=0.016173730442336543}, {"X"=9.49, "Y"=0.03054523744592707}, {"X"=9.5, "Y"=0.06893517436902041}, {"X"=9.51, "Y"=0.05646281391609046}, {"X"=9.52, "Y"=-0.059268731101496414}, {"X"=9.53, "Y"=-0.0005691525824747475}, {"X"=9.540000000000001, "Y"=-0.01685017360403408}, {"X"=9.55, "Y"=0.040007881874544515}, {"X"=9.56, "Y"=-0.06535008218683988}, {"X"=9.57, "Y"=0.06798698936257894}, {"X"=9.58, "Y"=-0.021774851376311286}, {"X"=9.59, "Y"=0.05058197790354009}, {"X"=9.6, "Y"=-0.006419807008853156}, {"X"=9.61, "Y"=-0.048280454361683954}, {"X"=9.620000000000001, "Y"=0.016279780403421137}, {"X"=9.63, "Y"=0.11502905845703057}, {"X"=9.64, "Y"=0.024969749298841937}, {"X"=9.65, "Y"=0.020719607062632338}, {"X"=9.66, "Y"=0.08613817965424753}, {"X"=9.67, "Y"=0.026451062270922712}, {"X"=9.68, "Y"=-0.011820728651824399}, {"X"=9.69, "Y"=-0.020879969277361077}, {"X"=9.700000000000001, "Y"=-0.008345465126225885}, {"X"=9.71, "Y"=0.034946933648476106}, {"X"=9.72, "Y"=0.044169962234250806}, {"X"=9.73, "Y"=-0.004055550980382885}, {"X"=9.74, "Y"=0.0033525416296074405}, {"X"=9.75, "Y"=0.06926918779214472}, {"X"=9.76, "Y"=-0.014601245128364507}, {"X"=9.77, "Y"=0.1100746716888515}, {"X"=9.78, "Y"=-0.020818296217770798}, {"X"=9.790000000000001, "Y"=0.0816722750384525}, {"X"=9.8, "Y"=0.046317409355601816}, {"X"=9.81, "Y"=0.005587329814392138}, {"X"=9.82, "Y"=-0.020665578337735524}, {"X"=9.83, "Y"=-0.009831477880200957}, {"X"=9.84, "Y"=-0.004473500514391083}, {"X"=9.85, "Y"=-0.020381152976647606}, {"X"=9.86, "Y"=0.03021476180719726}, {"X"=9.870000000000001, "Y"=0.030707656530512304}, {"X"=9.88, "Y"=0.005728359820610928}, {"X"=9.89, "Y"=-0.02690587170520143}, {"X"=9.9, "Y"=0.04431095765881365}, {"X"=9.91, "Y"=0.00933810755766251}, {"X"=9.92, "Y"=-0.021332572097527897}, {"X"=9.93, "Y"=0.04526925694831106}, {"X"=9.94, "Y"=0.002911768418863163}, {"X"=9.950000000000001, "Y"=-0.04603162133164909}, {"X"=9.96, "Y"=0.02552925716741984}, {"X"=9.97, "Y"=-0.008762302726763187}, {"X"=9.98, "Y"=-0.03754185096667118}, {"X"=9.99, "Y"=-0.002765561310605136}, {"X"=10.0, "Y"=0.01770546659436293}, {"X"=10.01, "Y"=-0.01823569279232122}, {"X"=10.02, "Y"=0.04340327637078868}, {"X"=10.03, "Y"=0.005540485606305972}, {"X"=10.040000000000001, "Y"=0.026685034359900665}, {"X"=10.05, "Y"=0.06548979568307589}, {"X"=10.06, "Y"=-0.014819012543646145}, {"X"=10.07, "Y"=-0.08755458791178711}, {"X"=10.08, "Y"=-0.015225591816426782}, {"X"=10.09, "Y"=0.10485771161833951}, {"X"=10.1, "Y"=-0.0995386070781505}, {"X"=10.11, "Y"=-0.03126162639212432}, {"X"=10.120000000000001, "Y"=-0.015212946192221272}, {"X"=10.13, "Y"=0.024406457602645544}, {"X"=10.14, "Y"=-0.004940913695625486}, {"X"=10.15, "Y"=0.008584548699998373}, {"X"=10.16, "Y"=-0.030825705410375406}, {"X"=10.17, "Y"=0.0628328269533071}, {"X"=10.18, "Y"=0.025236188232558056}, {"X"=10.19, "Y"=0.03889044298838836}, {"X"=10.200000000000001, "Y"=-0.0021986268324740814}, {"X"=10.21, "Y"=-0.04605771824775015}, {"X"=10.22, "Y"=-0.0013387941669840274}, {"X"=10.23, "Y"=-0.05500316094654892}, {"X"=10.24, "Y"=0.027896591749809446}, {"X"=10.25, "Y"=0.09850796364905598}, {"X"=10.26, "Y"=0.03234353528364816}, {"X"=10.27, "Y"=-0.002266301327758223}, {"X"=10.28, "Y"=-0.0492285343960151}, {"X"=10.290000000000001, "Y"=0.04152142285669232}, {"X"=10.3, "Y"=-0.06567369834048305}, {"X"=10.31, "Y"=0.009585126496442234}, {"X"=10.32, "Y"=-0.05164341741840146}, {"X"=10.33, "Y"=0.001423395359792367}, {"X"=10.34, "Y"=0.060304714780093596}, {"X"=10.35, "Y"=0.05327909528762588}, {"X"=10.36, "Y"=-0.0051949943817443545}, {"X"=10.370000000000001, "Y"=-0.04590271252135254}, {"X"=10.38, "Y"=-0.0034575315814277374}, {"X"=10.39, "Y"=-0.03880641496210472}, {"X"=10.4, "Y"=-0.02950390797795767}, {"X"=10.41, "Y"=-0.05464379938384025}, {"X"=10.42, "Y"=0.002277258429828693}, {"X"=10.43, "Y"=0.06617570890008787}, {"X"=10.44, "Y"=-0.08110744676155049}, {"X"=10.450000000000001, "Y"=0.020363840707663096}, {"X"=10.46, "Y"=0.03369411474841223}, {"X"=10.47, "Y"=-0.017388086277908416}, {"X"=10.48, "Y"=0.03773590410370819}, {"X"=10.49, "Y"=0.025096561508573468}, {"X"=10.5, "Y"=-0.009007463057025619}, {"X"=10.51, "Y"=-0.021628973389710166}, {"X"=10.52, "Y"=-0.030281377734130942}, {"X"=10.53, "Y"=-0.04760631067410149}, {"X"=10.540000000000001, "Y"=-0.024909355017102324}, {"X"=10.55, "Y"=-0.01977027827868364}, {"X"=10.56, "Y"=0.00867809547766562}, {"X"=10.57, "Y"=-0.025632604225037596}, {"X"=10.58, "Y"=-0.03391638802824602}, {"X"=10.59, "Y"=0.013100499414747828}, {"X"=10.6, "Y"=0.002059623454296871}, {"X"=10.61, "Y"=-0.03694933162106921}, {"X"=10.620000000000001, "Y"=0.035766028020107275}, {"X"=10.63, "Y"=-0.035139764886089345}, {"X"=10.64, "Y"=0.02878716180065135}, {"X"=10.65, "Y"=-0.011737233567594822}, {"X"=10.66, "Y"=-0.03381187374472419}, {"X"=10.67, "Y"=0.03302750158573598}, {"X"=10.68, "Y"=0.004210891976615795}, {"X"=10.69, "Y"=-0.00749881589708159}, {"X"=10.700000000000001, "Y"=-0.013766590187439125}, {"X"=10.71, "Y"=-0.03687625178165745}, {"X"=10.72, "Y"=0.032724089688411846}, {"X"=10.73, "Y"=-0.024644331511987912}, {"X"=10.74, "Y"=-0.053352977446023145}, {"X"=10.75, "Y"=0.02550748734665486}, {"X"=10.76, "Y"=0.010198188030605267}, {"X"=10.77, "Y"=-0.030612586608849583}, {"X"=10.78, "Y"=0.039427503583717785}, {"X"=10.790000000000001, "Y"=-0.025162468578579664}, {"X"=10.8, "Y"=0.02776195067825019}, {"X"=10.81, "Y"=-0.01603415873858073}, {"X"=10.82, "Y"=-0.06045769772469677}, {"X"=10.83, "Y"=0.025942325638020076}, {"X"=10.84, "Y"=0.004137847058915872}, {"X"=10.85, "Y"=-0.002863835001448388}, {"X"=10.86, "Y"=0.007505598341979914}, {"X"=10.870000000000001, "Y"=0.0031345146932761645}, {"X"=10.88, "Y"=-0.020659179011863614}, {"X"=10.89, "Y"=-0.04496596297943384}, {"X"=10.9, "Y"=0.017036783058339208}, {"X"=10.91, "Y"=0.007568938715797863}, {"X"=10.92, "Y"=0.022936081310774327}, {"X"=10.93, "Y"=0.006143183511386233}, {"X"=10.94, "Y"=0.054121457514090844}, {"X"=10.950000000000001, "Y"=0.026151886046193312}, {"X"=10.96, "Y"=-0.00978491551063483}, {"X"=10.97, "Y"=-0.021830146685051066}, {"X"=10.98, "Y"=-0.01839472656720117}, {"X"=10.99, "Y"=0.024077350957294883}, {"X"=11.0, "Y"=-0.038691682672640754}, {"X"=11.01, "Y"=0.027137073188565418}, {"X"=11.02, "Y"=0.0028456813694615495}, {"X"=11.03, "Y"=0.003115724505676395}, {"X"=11.040000000000001, "Y"=-0.04645145434699821}, {"X"=11.05, "Y"=-0.016823792201651238}, {"X"=11.06, "Y"=-0.021164592667862636}, {"X"=11.07, "Y"=0.07811440717928028}, {"X"=11.08, "Y"=-0.08731235726392031}, {"X"=11.09, "Y"=0.04471643223169786}, {"X"=11.1, "Y"=0.046316886818709005}, {"X"=11.11, "Y"=-0.0879564234413608}, {"X"=11.120000000000001, "Y"=0.014891186103125934}, {"X"=11.13, "Y"=-0.026879678522220563}, {"X"=11.14, "Y"=0.03429366253607521}, {"X"=11.15, "Y"=-0.09065761656318955}, {"X"=11.16, "Y"=0.026522338537293792}, {"X"=11.17, "Y"=-0.031210878304470422}, {"X"=11.18, "Y"=0.048311689224734805}, {"X"=11.19, "Y"=-0.025639421793051717}, {"X"=11.200000000000001, "Y"=-0.07783808743940933}, {"X"=11.21, "Y"=0.04188994037406393}, {"X"=11.22, "Y"=0.022140068414777996}, {"X"=11.23, "Y"=-3.4350972734204613e-06}, {"X"=11.24, "Y"=-0.015522238593157872}, {"X"=11.25, "Y"=-0.024437389788721134}, {"X"=11.26, "Y"=0.004119762041696057}, {"X"=11.27, "Y"=-0.03496353617180203}, {"X"=11.28, "Y"=0.03356737707660916}, {"X"=11.290000000000001, "Y"=-0.03893736708612916}, {"X"=11.3, "Y"=0.00840502925013949}, {"X"=11.31, "Y"=0.03508695574852237}, {"X"=11.32, "Y"=-0.02524156569651407}, {"X"=11.33, "Y"=-0.014961438761217884}, {"X"=11.34, "Y"=0.016294077319294525}, {"X"=11.35, "Y"=-0.042756751106938246}, {"X"=11.36, "Y"=-0.07170391296700386}, {"X"=11.370000000000001, "Y"=0.03799620182294604}, {"X"=11.38, "Y"=-0.07394555195106417}, {"X"=11.39, "Y"=0.023332176253058882}, {"X"=11.4, "Y"=0.01120046492607502}, {"X"=11.41, "Y"=0.07127444009272133}, {"X"=11.42, "Y"=-0.046969316539414385}, {"X"=11.43, "Y"=-0.06814083027553307}, {"X"=11.44, "Y"=-0.017276938447451252}, {"X"=11.450000000000001, "Y"=0.07128198007003361}, {"X"=11.46, "Y"=-0.053048705065121535}, {"X"=11.47, "Y"=0.01728987848169969}, {"X"=11.48, "Y"=-0.023182322539294094}, {"X"=11.49, "Y"=0.06618397619630906}, {"X"=11.5, "Y"=0.04674630169291535}, {"X"=11.51, "Y"=-0.04431180895545657}, {"X"=11.52, "Y"=-0.018911887095203084}, {"X"=11.53, "Y"=0.04522909683413552}, {"X"=11.540000000000001, "Y"=0.030716142343467572}, {"X"=11.55, "Y"=0.019392993702691305}, {"X"=11.56, "Y"=0.009339726546956646}, {"X"=11.57, "Y"=0.00197477712690502}, {"X"=11.58, "Y"=-0.08584435860686317}, {"X"=11.59, "Y"=-0.004186667037945143}, {"X"=11.6, "Y"=-0.002752604974430146}, {"X"=11.61, "Y"=-0.03300562622822459}, {"X"=11.620000000000001, "Y"=-0.001698092269283985}, {"X"=11.63, "Y"=-0.0021659191736056183}, {"X"=11.64, "Y"=-0.012913141144447358}, {"X"=11.65, "Y"=-0.012443392886870581}, {"X"=11.66, "Y"=-0.01984314579033621}, {"X"=11.67, "Y"=0.014573039788753765}, {"X"=11.68, "Y"=-0.03769160343372623}, {"X"=11.69, "Y"=-0.0056929626243671936}, {"X"=11.700000000000001, "Y"=-0.06170024766768535}, {"X"=11.71, "Y"=-0.006932390471670644}, {"X"=11.72, "Y"=-0.011282369189319361}, {"X"=11.73, "Y"=0.009910387139199835}, {"X"=11.74, "Y"=0.015675844128213632}, {"X"=11.75, "Y"=0.06144142274908255}, {"X"=11.76, "Y"=0.04814676004941874}, {"X"=11.77, "Y"=-0.01970473414740711}, {"X"=11.78, "Y"=0.03873284953451401}, {"X"=11.790000000000001, "Y"=-0.05468495603171127}, {"X"=11.8, "Y"=0.03586958983136579}, {"X"=11.81, "Y"=-0.061203928497406496}, {"X"=11.82, "Y"=-0.015476791366711932}, {"X"=11.83, "Y"=0.038250738157126395}, {"X"=11.84, "Y"=0.017505992646566503}, {"X"=11.85, "Y"=0.0206403268297335}, {"X"=11.86, "Y"=-0.04058414851936508}, {"X"=11.870000000000001, "Y"=0.03284444260192616}, {"X"=11.88, "Y"=-0.028882263863599246}, {"X"=11.89, "Y"=-0.00603850410897971}, {"X"=11.9, "Y"=-0.016902698325479974}, {"X"=11.91, "Y"=-0.008515681529121289}, {"X"=11.92, "Y"=0.055666655361718956}, {"X"=11.93, "Y"=-0.07015681100345497}, {"X"=11.94, "Y"=0.01446437616335776}, {"X"=11.950000000000001, "Y"=-0.029316819640390616}, {"X"=11.96, "Y"=-0.017756205102601046}, {"X"=11.97, "Y"=-0.014353024655789543}, {"X"=11.98, "Y"=-0.01691291077898154}, {"X"=11.99, "Y"=-0.03278269768589884}, {"X"=12.0, "Y"=-0.03732920966914033}, {"X"=12.01, "Y"=-0.01177901850686184}, {"X"=12.02, "Y"=-0.03334621378407613}, {"X"=12.03, "Y"=-0.005551195803171373}, {"X"=12.040000000000001, "Y"=-0.03963902477300333}, {"X"=12.05, "Y"=-0.015594962628123273}, {"X"=12.06, "Y"=-0.054548476738995696}, {"X"=12.07, "Y"=0.048968784785045086}, {"X"=12.08, "Y"=0.019101845290804272}, {"X"=12.09, "Y"=0.009955022165978765}, {"X"=12.1, "Y"=-0.06016323456901181}, {"X"=12.11, "Y"=-0.03986290976644216}, {"X"=12.120000000000001, "Y"=-0.06489763591660393}, {"X"=12.13, "Y"=-0.014330499931071949}, {"X"=12.14, "Y"=0.005793816340324286}, {"X"=12.15, "Y"=-0.003675051035752876}, {"X"=12.16, "Y"=0.03406156516405164}, {"X"=12.17, "Y"=0.037279640773147736}, {"X"=12.18, "Y"=-0.0034383935021712205}, {"X"=12.19, "Y"=0.029561803080611453}, {"X"=12.200000000000001, "Y"=-0.020267120306489698}, {"X"=12.21, "Y"=-0.0026343425601580614}, {"X"=12.22, "Y"=0.05295696668049416}, {"X"=12.23, "Y"=0.05829985956167025}, {"X"=12.24, "Y"=0.028641417762388925}, {"X"=12.25, "Y"=-0.019289956523570986}, {"X"=12.26, "Y"=-0.002108373340663832}, {"X"=12.27, "Y"=0.06163780034509168}, {"X"=12.28, "Y"=0.04553774196924483}, {"X"=12.290000000000001, "Y"=-0.0011847755686442702}, {"X"=12.3, "Y"=-0.00045588406828503305}, {"X"=12.31, "Y"=0.003941580506834152}, {"X"=12.32, "Y"=0.04820396742483423}, {"X"=12.33, "Y"=-0.039930167688576705}, {"X"=12.34, "Y"=0.03421348789301834}, {"X"=12.35, "Y"=-0.009135153283816635}, {"X"=12.36, "Y"=0.042925316211976}, {"X"=12.370000000000001, "Y"=-0.06330566129109677}, {"X"=12.38, "Y"=0.046768873177908156}, {"X"=12.39, "Y"=0.0304997650308929}, {"X"=12.4, "Y"=0.021506084787063267}, {"X"=12.41, "Y"=-0.045645407317517483}, {"X"=12.42, "Y"=-0.01806971311544316}, {"X"=12.43, "Y"=0.03045145573801973}, {"X"=12.44, "Y"=0.08406334805168615}, {"X"=12.450000000000001, "Y"=0.06738061289920252}, {"X"=12.46, "Y"=-0.0457409991310705}, {"X"=12.47, "Y"=0.06275415937784284}, {"X"=12.48, "Y"=0.06774390116514886}, {"X"=12.49, "Y"=0.08835818434920617}, {"X"=12.5, "Y"=0.07305300141851373}, {"X"=12.51, "Y"=-0.059196957326604904}, {"X"=12.52, "Y"=-0.0007531783013525338}, {"X"=12.53, "Y"=-0.005024643636508983}, {"X"=12.540000000000001, "Y"=0.03501009803913044}, {"X"=12.55, "Y"=-0.03631800290386857}, {"X"=12.56, "Y"=0.05512585019821699}, {"X"=12.57, "Y"=-0.03167301392879023}, {"X"=12.58, "Y"=0.02134082326453196}, {"X"=12.59, "Y"=-0.03494889608333539}, {"X"=12.6, "Y"=-0.007631505216622949}, {"X"=12.61, "Y"=-0.00041857580175074606}, {"X"=12.620000000000001, "Y"=-0.004917213350073705}, {"X"=12.63, "Y"=0.021066462932331276}, {"X"=12.64, "Y"=0.003912018568992143}, {"X"=12.65, "Y"=0.01860948180484933}, {"X"=12.66, "Y"=0.009696906991288145}, {"X"=12.67, "Y"=0.010813948850511592}, {"X"=12.68, "Y"=0.03321008165227003}, {"X"=12.69, "Y"=-0.06010871524132325}, {"X"=12.700000000000001, "Y"=-0.020387044883574866}, {"X"=12.71, "Y"=-0.002192407631732779}, {"X"=12.72, "Y"=0.0006765434179596893}, {"X"=12.73, "Y"=-0.04541487374609964}, {"X"=12.74, "Y"=-0.08631142602905262}, {"X"=12.75, "Y"=0.03450032985300276}, {"X"=12.76, "Y"=-0.00967147677122238}, {"X"=12.77, "Y"=-0.05110673648989831}, {"X"=12.78, "Y"=0.042072225791115136}, {"X"=12.790000000000001, "Y"=0.03976601989184078}, {"X"=12.8, "Y"=-0.05512406818322855}, {"X"=12.81, "Y"=-0.06836424071523382}, {"X"=12.82, "Y"=-0.049159792777060014}, {"X"=12.83, "Y"=-0.007345466108714687}, {"X"=12.84, "Y"=0.07270442704248417}, {"X"=12.85, "Y"=0.06424837186771548}, {"X"=12.86, "Y"=-0.03418102457611166}, {"X"=12.870000000000001, "Y"=0.05828247519539988}, {"X"=12.88, "Y"=0.061978403551360195}, {"X"=12.89, "Y"=-0.0530620683683963}, {"X"=12.9, "Y"=0.01776818267458486}, {"X"=12.91, "Y"=0.022730839883998818}, {"X"=12.92, "Y"=0.0013179979894771014}, {"X"=12.93, "Y"=-0.03328590738791486}, {"X"=12.94, "Y"=0.024821233062040756}, {"X"=12.950000000000001, "Y"=0.025315535858369147}, {"X"=12.96, "Y"=0.026953763905769815}, {"X"=12.97, "Y"=0.008152064824681775}, {"X"=12.98, "Y"=-0.006447164111000234}, {"X"=12.99, "Y"=-0.023049463260470235}, {"X"=13.0, "Y"=0.03147172694864609}, {"X"=13.01, "Y"=-0.023872952895644554}, {"X"=13.02, "Y"=-0.025786086538264474}, {"X"=13.030000000000001, "Y"=-0.021396894088345095}, {"X"=13.040000000000001, "Y"=-0.03547103584776813}, {"X"=13.05, "Y"=0.013944657985473403}, {"X"=13.06, "Y"=0.03804005672643368}, {"X"=13.07, "Y"=-0.04046639064243082}, {"X"=13.08, "Y"=0.026160560140255473}, {"X"=13.09, "Y"=-0.007497888817411162}, {"X"=13.1, "Y"=-0.007891728453690901}, {"X"=13.11, "Y"=-0.013210377251319353}, {"X"=13.120000000000001, "Y"=0.06138387766849904}, {"X"=13.13, "Y"=-0.0037675068951529356}, {"X"=13.14, "Y"=-0.06450650248675338}, {"X"=13.15, "Y"=0.04557865493720039}, {"X"=13.16, "Y"=0.021961987352317407}, {"X"=13.17, "Y"=0.023235682231499858}, {"X"=13.18, "Y"=0.04562994309718373}, {"X"=13.19, "Y"=-0.05929192621767834}, {"X"=13.200000000000001, "Y"=-0.03205913431694592}, {"X"=13.21, "Y"=-0.007211160924753355}, {"X"=13.22, "Y"=-0.03875206722341212}, {"X"=13.23, "Y"=0.024013502035423996}, {"X"=13.24, "Y"=-0.042947657411393635}, {"X"=13.25, "Y"=-0.05077619169012759}, {"X"=13.26, "Y"=0.013916399077172403}, {"X"=13.27, "Y"=-0.047042831553449176}, {"X"=13.280000000000001, "Y"=0.04879092354453138}, {"X"=13.290000000000001, "Y"=0.044713718012742765}, {"X"=13.3, "Y"=0.0030379988474894507}, {"X"=13.31, "Y"=0.012533431506854733}, {"X"=13.32, "Y"=-0.05163527123667702}, {"X"=13.33, "Y"=0.025870894929929805}, {"X"=13.34, "Y"=-0.04585027228193244}, {"X"=13.35, "Y"=0.0650334447677042}, {"X"=13.36, "Y"=-0.04988234539966267}, {"X"=13.370000000000001, "Y"=0.06189027326789377}, {"X"=13.38, "Y"=-0.05747446762770939}, {"X"=13.39, "Y"=0.07968268997134374}, {"X"=13.4, "Y"=0.07478210793465907}, {"X"=13.41, "Y"=-0.03499319459692414}, {"X"=13.42, "Y"=0.014411009158007446}, {"X"=13.43, "Y"=-0.019528088303460873}, {"X"=13.44, "Y"=0.04033733025399785}, {"X"=13.450000000000001, "Y"=0.007187227995287849}, {"X"=13.46, "Y"=-0.005319217566302042}, {"X"=13.47, "Y"=0.020791364850032554}, {"X"=13.48, "Y"=0.0264007191542497}, {"X"=13.49, "Y"=0.006224795120981209}, {"X"=13.5, "Y"=-0.025487138753824433}, {"X"=13.51, "Y"=-0.0579204699014544}, {"X"=13.52, "Y"=0.03312523177980121}, {"X"=13.530000000000001, "Y"=-0.02041488071413103}, {"X"=13.540000000000001, "Y"=0.0549277275403148}, {"X"=13.55, "Y"=0.0584778839341155}, {"X"=13.56, "Y"=-0.0032254876948123244}, {"X"=13.57, "Y"=-0.010054546147753534}, {"X"=13.58, "Y"=0.010475361686996186}, {"X"=13.59, "Y"=-0.018233524374685096}, {"X"=13.6, "Y"=-0.022964499838674827}, {"X"=13.61, "Y"=-0.03317283948874555}, {"X"=13.620000000000001, "Y"=0.0293908042528409}, {"X"=13.63, "Y"=0.027379211064498005}, {"X"=13.64, "Y"=0.011308226790791864}, {"X"=13.65, "Y"=0.017199211119020206}, {"X"=13.66, "Y"=0.032971881060425534}, {"X"=13.67, "Y"=-0.01105410605026735}, {"X"=13.68, "Y"=-0.024356688336625576}, {"X"=13.69, "Y"=0.04384569914683373}, {"X"=13.700000000000001, "Y"=-0.03799016553244929}, {"X"=13.71, "Y"=-0.047600759177065646}, {"X"=13.72, "Y"=0.013148865817900847}, {"X"=13.73, "Y"=-0.007519795923847024}, {"X"=13.74, "Y"=0.0280983225547749}, {"X"=13.75, "Y"=-0.003794838411298647}, {"X"=13.76, "Y"=-0.00033346181135394866}, {"X"=13.77, "Y"=-0.017476425691065202}, {"X"=13.780000000000001, "Y"=9.600100841411223e-05}, {"X"=13.790000000000001, "Y"=0.006474751500845208}, {"X"=13.8, "Y"=0.002249581112273856}, {"X"=13.81, "Y"=0.011051544837183881}, {"X"=13.82, "Y"=0.004806920475840161}, {"X"=13.83, "Y"=-0.0028611162056599903}, {"X"=13.84, "Y"=-0.03248879219399819}, {"X"=13.85, "Y"=0.0181922727046812}, {"X"=13.86, "Y"=0.0177683358130373}, {"X"=13.870000000000001, "Y"=-0.025055865046079526}, {"X"=13.88, "Y"=0.005151810295689467}, {"X"=13.89, "Y"=0.03818841805077669}, {"X"=13.9, "Y"=-0.02629199968903845}, {"X"=13.91, "Y"=-0.0057592936154600115}, {"X"=13.92, "Y"=-0.010971224227720452}, {"X"=13.93, "Y"=-0.015049046478532587}, {"X"=13.94, "Y"=-0.010550822850039058}, {"X"=13.950000000000001, "Y"=-0.00871670575285426}, {"X"=13.96, "Y"=0.009399789168500827}, {"X"=13.97, "Y"=-0.0006942242907500836}, {"X"=13.98, "Y"=-0.0007274645760458175}, {"X"=13.99, "Y"=0.014946538709524948}, {"X"=14.0, "Y"=-0.02455943389950946}, {"X"=14.01, "Y"=-0.014069359155782595}, {"X"=14.02, "Y"=0.0026385152492742828}, {"X"=14.030000000000001, "Y"=-0.003265708029176648}, {"X"=14.040000000000001, "Y"=-0.0012488372748498684}, {"X"=14.05, "Y"=-0.006760783589437174}, {"X"=14.06, "Y"=0.016835401111766898}, {"X"=14.07, "Y"=-0.005207843278839425}, {"X"=14.08, "Y"=-0.0019950389444577015}, {"X"=14.09, "Y"=-0.002699848863933962}, {"X"=14.1, "Y"=0.013950855756684375}, {"X"=14.11, "Y"=-0.015864561602368966}, {"X"=14.120000000000001, "Y"=-0.004083002951314334}, {"X"=14.13, "Y"=-0.004273302138415809}, {"X"=14.14, "Y"=-0.0018909821006941824}, {"X"=14.15, "Y"=-0.0004862564366754003}, {"X"=14.16, "Y"=-0.001496101488253494}, {"X"=14.17, "Y"=6.323797641276233e-05}, {"X"=14.18, "Y"=-0.0101419246775405}, {"X"=14.19, "Y"=-0.0008505435719848785}, {"X"=14.200000000000001, "Y"=0.0006575937867088575}, {"X"=14.21, "Y"=-0.00040939996508086165}, {"X"=14.22, "Y"=-0.003943972732149462}, {"X"=14.23, "Y"=-0.006598659215288691}, {"X"=14.24, "Y"=0.0011228771971995113}, {"X"=14.25, "Y"=-0.00254264603801796}, {"X"=14.26, "Y"=-0.001442708126234226}, {"X"=14.27, "Y"=0.0072880196733293556}, {"X"=14.280000000000001, "Y"=-0.0017269396956604225}, {"X"=14.290000000000001, "Y"=-0.003991513947316387}, {"X"=14.3, "Y"=0.0019653407531636372}, {"X"=14.31, "Y"=-0.00011219082014665359}, {"X"=14.32, "Y"=0.002513144643025705}, {"X"=14.33, "Y"=-0.004335450251149183}, {"X"=14.34, "Y"=-0.005448650397533076}, {"X"=14.35, "Y"=-0.002325504633719153}, {"X"=14.36, "Y"=-0.0003577750443843427}, {"X"=14.370000000000001, "Y"=-0.00011020810345934066}, {"X"=14.38, "Y"=0.0004509790785101307}, {"X"=14.39, "Y"=0.00021850187902758235}, {"X"=14.4, "Y"=0.0017154583706670773}, {"X"=14.41, "Y"=0.0002204269787434222}, {"X"=14.42, "Y"=0.0016910141534926375}, {"X"=14.43, "Y"=0.0030276852800448077}, {"X"=14.44, "Y"=0.0012447419203249273}, {"X"=14.450000000000001, "Y"=-0.0004886007033891023}, {"X"=14.46, "Y"=0.0018275989368584354}, {"X"=14.47, "Y"=-0.003399204839451616}, {"X"=14.48, "Y"=-0.003929338923548843}, {"X"=14.49, "Y"=0.0023248099159120473}, {"X"=14.5, "Y"=-0.0009133865004980419}, {"X"=14.51, "Y"=0.0028594909049350827}, {"X"=14.52, "Y"=0.0005417817500901893}, {"X"=14.530000000000001, "Y"=-0.0011368245196488821}, {"X"=14.540000000000001, "Y"=0.0018394066143917788}, {"X"=14.55, "Y"=0.0021731113769384606}, {"X"=14.56, "Y"=-0.0025240787910780697}, {"X"=14.57, "Y"=0.0005551970016141645}, {"X"=14.58, "Y"=-0.00037134052226804213}, {"X"=14.59, "Y"=0.0016525999857394536}, {"X"=14.6, "Y"=0.0016120988974921045}, {"X"=14.61, "Y"=0.00017968077077439417}, {"X"=14.620000000000001, "Y"=0.0007011826377636738}, {"X"=14.63, "Y"=-0.0013246110925769147}, {"X"=14.64, "Y"=0.0036981442141883476}, {"X"=14.65, "Y"=-0.0006677552977572203}, {"X"=14.66, "Y"=-0.001604469321058006}, {"X"=14.67, "Y"=6.418480586717012e-05}, {"X"=14.68, "Y"=-0.002233094526130234}, {"X"=14.69, "Y"=-0.0007056314203200298}, {"X"=14.700000000000001, "Y"=-0.0030885077653608696}, {"X"=14.71, "Y"=0.001767429830534229}, {"X"=14.72, "Y"=-0.002717960943999489}, {"X"=14.73, "Y"=0.0019145183936858773}, {"X"=14.74, "Y"=-0.0010128807172597558}, {"X"=14.75, "Y"=0.002861756020693669}, {"X"=14.76, "Y"=0.0001343020024642306}, {"X"=14.77, "Y"=-0.003130215561734028}, {"X"=14.780000000000001, "Y"=0.001611298015056677}, {"X"=14.790000000000001, "Y"=0.006374054861190942}, {"X"=14.8, "Y"=-0.00036700289634934144}, {"X"=14.81, "Y"=7.973390422958093e-05}, {"X"=14.82, "Y"=-0.0009520284786784307}, {"X"=14.83, "Y"=0.001962849968291908}, {"X"=14.84, "Y"=0.0003697790001736182}, {"X"=14.85, "Y"=-0.005039611268780405}, {"X"=14.86, "Y"=0.001733362662562592}, {"X"=14.870000000000001, "Y"=-0.00333947676415528}, {"X"=14.88, "Y"=-0.003524941230785992}, {"X"=14.89, "Y"=-0.004738716866774193}, {"X"=14.9, "Y"=0.002894058898669759}, {"X"=14.91, "Y"=-0.003348817159431168}, {"X"=14.92, "Y"=-0.0018839486012317832}, {"X"=14.93, "Y"=0.0012264793781274783}, {"X"=14.94, "Y"=-0.010473364284054432}, {"X"=14.950000000000001, "Y"=-0.00032062690167519}, {"X"=14.96, "Y"=0.002599663387836571}, {"X"=14.97, "Y"=0.0031070632752323397}, {"X"=14.98, "Y"=0.003847340053560494}, {"X"=14.99, "Y"=0.007136433172382958}, {"X"=15.0, "Y"=-0.002337693018177515}, {"X"=15.01, "Y"=-0.010947521569919443}, {"X"=15.02, "Y"=0.010529930394911147}, {"X"=15.030000000000001, "Y"=0.007515309843907739}, {"X"=15.040000000000001, "Y"=0.008565442256893749}, {"X"=15.05, "Y"=0.015437259497443973}, {"X"=15.06, "Y"=-0.012102791298031844}, {"X"=15.07, "Y"=-0.027997373241051417}, {"X"=15.08, "Y"=-0.06735651482403204}, {"X"=15.09, "Y"=-0.010087221383069526}, {"X"=15.1, "Y"=0.019405397178850026}, {"X"=15.11, "Y"=0.01458703839445437}, {"X"=15.120000000000001, "Y"=-0.009563428808444933}, {"X"=15.13, "Y"=0.0022210923177704844}, {"X"=15.14, "Y"=-0.002207257236245975}, {"X"=15.15, "Y"=-0.017819407333784273}, {"X"=15.16, "Y"=0.01582596220964018}, {"X"=15.17, "Y"=0.032034091983081346}, {"X"=15.18, "Y"=-0.001625729535482353}, {"X"=15.19, "Y"=0.003887172629912977}, {"X"=15.200000000000001, "Y"=0.003967643861074346}, {"X"=15.21, "Y"=-0.006840310765020067}, {"X"=15.22, "Y"=-0.0018403229425266278}, {"X"=15.23, "Y"=-0.006633766578828823}, {"X"=15.24, "Y"=0.015738153495578985}, {"X"=15.25, "Y"=-0.0011601672088361681}, {"X"=15.26, "Y"=0.012140194303375427}, {"X"=15.27, "Y"=0.009640209648819072}, {"X"=15.280000000000001, "Y"=-0.004882749510748431}, {"X"=15.290000000000001, "Y"=0.007068064983754778}, {"X"=15.3, "Y"=0.017845706821971917}, {"X"=15.31, "Y"=0.0009656719750415429}, {"X"=15.32, "Y"=0.009648552148518567}, {"X"=15.33, "Y"=-0.009605102062915115}, {"X"=15.34, "Y"=0.03074163680759208}, {"X"=15.35, "Y"=0.0013559989979730182}, {"X"=15.36, "Y"=0.0011971133601929634}, {"X"=15.370000000000001, "Y"=0.0008987659567042187}, {"X"=15.38, "Y"=0.00012052575305205283}, {"X"=15.39, "Y"=-0.00042864372175281445}, {"X"=15.4, "Y"=-0.0024918840570961388}, {"X"=15.41, "Y"=-0.0009098792291340196}, {"X"=15.42, "Y"=0.0025844157833174227}, {"X"=15.43, "Y"=0.0011658598887255814}, {"X"=15.44, "Y"=0.0015546286139359344}, {"X"=15.450000000000001, "Y"=-1.5474165816059472e-05}, {"X"=15.46, "Y"=0.00018164108103266297}, {"X"=15.47, "Y"=-0.0021431776027606153}, {"X"=15.48, "Y"=0.0016233790747037025}, {"X"=15.49, "Y"=-0.0005731522451201784}, {"X"=15.5, "Y"=-0.002343611710804925}, {"X"=15.51, "Y"=0.001307326366450474}, {"X"=15.52, "Y"=6.52084724984878e-05}, {"X"=15.530000000000001, "Y"=0.0011355003001370018}, {"X"=15.540000000000001, "Y"=-0.0036476334692636028}, {"X"=15.55, "Y"=-0.007027350933141588}, {"X"=15.56, "Y"=0.0030072301126117884}, {"X"=15.57, "Y"=9.727280085488776e-05}, {"X"=15.58, "Y"=-0.006539341897252311}, {"X"=15.59, "Y"=-0.005889536313141117}, {"X"=15.6, "Y"=0.012558949038533546}, {"X"=15.61, "Y"=0.014567763628138282}, {"X"=15.620000000000001, "Y"=0.0016683390727731875}, {"X"=15.63, "Y"=-0.003207269198200286}, {"X"=15.64, "Y"=0.0109361062747638}, {"X"=15.65, "Y"=0.020813766474362113}, {"X"=15.66, "Y"=0.015761795747180236}, {"X"=15.67, "Y"=0.009966655762278193}, {"X"=15.68, "Y"=-0.01346981660489105}, {"X"=15.69, "Y"=0.025930470819653766}, {"X"=15.700000000000001, "Y"=-0.00966438913466323}, {"X"=15.71, "Y"=0.007293522296163396}, {"X"=15.72, "Y"=0.0036084050754574843}, {"X"=15.73, "Y"=0.017483593355438927}, {"X"=15.74, "Y"=0.01884598105454788}, {"X"=15.75, "Y"=0.006216488909514107}, {"X"=15.76, "Y"=0.013555272488527361}, {"X"=15.77, "Y"=0.016385273802036603}, {"X"=15.780000000000001, "Y"=0.01710120615694242}, {"X"=15.790000000000001, "Y"=0.013723344556712607}, {"X"=15.8, "Y"=0.002662168817237957}, {"X"=15.81, "Y"=0.016325862935341256}, {"X"=15.82, "Y"=-0.013162430019579943}, {"X"=15.83, "Y"=0.008002501767185744}, {"X"=15.84, "Y"=-0.009070116486842495}, {"X"=15.85, "Y"=0.007857191197247568}, {"X"=15.86, "Y"=0.012205455665622849}, {"X"=15.870000000000001, "Y"=-0.004254402358135283}, {"X"=15.88, "Y"=-0.0015693059335765915}, {"X"=15.89, "Y"=-0.009547895967213092}, {"X"=15.9, "Y"=-0.009769746324011888}, {"X"=15.91, "Y"=-0.012237638099846496}, {"X"=15.92, "Y"=0.016735440801458282}, {"X"=15.93, "Y"=-0.0352473846593053}, {"X"=15.94, "Y"=0.02287379013163973}, {"X"=15.950000000000001, "Y"=0.012164641171252894}, {"X"=15.96, "Y"=-0.0035099852184367706}, {"X"=15.97, "Y"=0.008709100599056314}, {"X"=15.98, "Y"=0.031055241317594056}, {"X"=15.99, "Y"=0.009116986605221755}, {"X"=16.0, "Y"=-0.05408814329901362}, {"X"=16.009999999999998, "Y"=-0.004483070094855689}, {"X"=16.02, "Y"=0.026715227771723252}, {"X"=16.03, "Y"=0.0074866499826397115}, {"X"=16.04, "Y"=-0.013024417244190074}, {"X"=16.05, "Y"=0.012553482230388949}, {"X"=16.060000000000002, "Y"=0.0007882891383665107}, {"X"=16.07, "Y"=0.008350991635816632}, {"X"=16.08, "Y"=-0.04854722805353287}, {"X"=16.09, "Y"=-0.013604386966066057}, {"X"=16.1, "Y"=0.0032264900672649846}, {"X"=16.11, "Y"=0.007508482218478601}, {"X"=16.12, "Y"=-0.006871883142913329}, {"X"=16.130000000000003, "Y"=0.013165555460390712}, {"X"=16.14, "Y"=-0.026090807028828558}, {"X"=16.15, "Y"=0.02495871362993808}, {"X"=16.16, "Y"=0.019583655886960427}, {"X"=16.17, "Y"=0.011267525737216746}, {"X"=16.18, "Y"=-0.01655761425614314}, {"X"=16.189999999999998, "Y"=0.015067199976860575}, {"X"=16.200000000000003, "Y"=-0.03806484220029106}, {"X"=16.21, "Y"=0.04868039465031352}, {"X"=16.22, "Y"=-0.04212386303563878}, {"X"=16.23, "Y"=0.0033227014711117134}, {"X"=16.240000000000002, "Y"=0.003305476826487954}, {"X"=16.25, "Y"=-0.017760092394150925}, {"X"=16.259999999999998, "Y"=0.014074692968495627}, {"X"=16.27, "Y"=0.009612264420210997}, {"X"=16.28, "Y"=0.029274031331923626}, {"X"=16.29, "Y"=0.03042508498552329}, {"X"=16.3, "Y"=-0.04695918800701697}, {"X"=16.310000000000002, "Y"=-0.018286795364806516}, {"X"=16.32, "Y"=-0.01828817401590632}, {"X"=16.33, "Y"=-0.020773362306667896}, {"X"=16.34, "Y"=-0.005623808462409614}, {"X"=16.35, "Y"=0.021004656068880946}, {"X"=16.36, "Y"=0.009650064658715828}, {"X"=16.37, "Y"=-0.015215886461990378}, {"X"=16.380000000000003, "Y"=0.025946308699344084}, {"X"=16.39, "Y"=0.0018330235718481036}, {"X"=16.4, "Y"=0.03344422748930816}, {"X"=16.41, "Y"=0.010634587491689312}, {"X"=16.42, "Y"=0.00018100793027547163}, {"X"=16.43, "Y"=-0.0052776599969199586}, {"X"=16.439999999999998, "Y"=-0.005410487781764517}, {"X"=16.450000000000003, "Y"=-0.014269689282542833}, {"X"=16.46, "Y"=-0.01230576129093669}, {"X"=16.47, "Y"=-0.021334139486109682}, {"X"=16.48, "Y"=0.010702417935340958}, {"X"=16.490000000000002, "Y"=0.015311694087533868}, {"X"=16.5, "Y"=0.0008656978786185776}, {"X"=16.509999999999998, "Y"=0.0350418916249582}, {"X"=16.52, "Y"=0.015324075567370997}, {"X"=16.53, "Y"=0.02110535609248051}, {"X"=16.54, "Y"=-0.01429167287661389}, {"X"=16.55, "Y"=-0.019855033011423197}, {"X"=16.560000000000002, "Y"=0.043445640070263636}, {"X"=16.57, "Y"=-0.025737602502018647}, {"X"=16.58, "Y"=0.015130422173997689}, {"X"=16.59, "Y"=0.015553476885662918}, {"X"=16.6, "Y"=-0.009511394687946663}, {"X"=16.61, "Y"=-0.0019149540861731012}, {"X"=16.62, "Y"=-0.0031127089578046486}, {"X"=16.630000000000003, "Y"=0.03635109328172618}, {"X"=16.64, "Y"=0.012139580269245054}, {"X"=16.65, "Y"=0.012619707554837881}, {"X"=16.66, "Y"=-0.033830941350182}, {"X"=16.67, "Y"=0.023646313845004215}, {"X"=16.68, "Y"=-0.03986146471931698}, {"X"=16.689999999999998, "Y"=-0.01728275006040665}, {"X"=16.700000000000003, "Y"=0.021144234250638216}, {"X"=16.71, "Y"=-0.012425238992114262}, {"X"=16.72, "Y"=-0.06086650692037046}, {"X"=16.73, "Y"=0.013998807559400608}, {"X"=16.740000000000002, "Y"=0.01604507859689541}, {"X"=16.75, "Y"=0.008961510880626637}, {"X"=16.759999999999998, "Y"=-0.013055413707098817}, {"X"=16.77, "Y"=-0.022114467784934706}, {"X"=16.78, "Y"=-0.008176348394686922}, {"X"=16.79, "Y"=0.041624431888648804}, {"X"=16.8, "Y"=0.0016806133071263357}, {"X"=16.810000000000002, "Y"=-0.01902164347051928}, {"X"=16.82, "Y"=0.001535302025812253}, {"X"=16.83, "Y"=0.008764028462232402}, {"X"=16.84, "Y"=0.017012919341742292}, {"X"=16.85, "Y"=0.0022868917124736887}, {"X"=16.86, "Y"=0.016487251750000435}, {"X"=16.87, "Y"=-0.01896203223878171}, {"X"=16.880000000000003, "Y"=0.016215345783807917}, {"X"=16.89, "Y"=-0.04287913853064131}, {"X"=16.9, "Y"=-0.02090686384761116}, {"X"=16.91, "Y"=0.008947732058980884}, {"X"=16.92, "Y"=0.010335940506983582}, {"X"=16.93, "Y"=0.010221730064136375}, {"X"=16.939999999999998, "Y"=0.014535730280744837}, {"X"=16.950000000000003, "Y"=0.002569548366792989}, {"X"=16.96, "Y"=-0.033644035159174586}, {"X"=16.97, "Y"=-0.02748784972730281}, {"X"=16.98, "Y"=0.019452378259028895}, {"X"=16.990000000000002, "Y"=-0.038741635711961465}, {"X"=17.0, "Y"=0.006263886588524989}, {"X"=17.01, "Y"=-0.008907333127364383}, {"X"=17.02, "Y"=0.0065152607927423944}, {"X"=17.03, "Y"=0.014190971431855435}, {"X"=17.04, "Y"=0.034649608971034765}, {"X"=17.05, "Y"=0.019979124419228535}, {"X"=17.06, "Y"=-0.022210735942466482}, {"X"=17.07, "Y"=0.04015373121143261}, {"X"=17.080000000000002, "Y"=-0.016878321015540244}, {"X"=17.09, "Y"=0.010881048869738317}, {"X"=17.1, "Y"=0.029381589845195333}, {"X"=17.11, "Y"=0.00999001119445144}, {"X"=17.12, "Y"=0.009726586158640969}, {"X"=17.13, "Y"=-0.06296281341261417}, {"X"=17.14, "Y"=0.012906157488000034}, {"X"=17.15, "Y"=0.010097575954164308}, {"X"=17.16, "Y"=-0.0037166174368025847}, {"X"=17.17, "Y"=0.018791922785169328}, {"X"=17.18, "Y"=0.03875550530914547}, {"X"=17.19, "Y"=-0.001886422391646934}, {"X"=17.2, "Y"=0.005086773473327167}, {"X"=17.21, "Y"=-0.019985628019680554}, {"X"=17.22, "Y"=0.02892595530889306}, {"X"=17.23, "Y"=-0.023183468501624355}, {"X"=17.240000000000002, "Y"=0.006914922201229171}, {"X"=17.25, "Y"=0.003490231411632234}, {"X"=17.26, "Y"=-0.0007616802224468342}, {"X"=17.27, "Y"=0.023569832082329448}, {"X"=17.28, "Y"=0.007974759100910545}, {"X"=17.29, "Y"=0.030595923796457314}, {"X"=17.3, "Y"=0.0038281766017609106}, {"X"=17.31, "Y"=0.0055478371188310924}, {"X"=17.32, "Y"=0.020608350259930783}, {"X"=17.330000000000002, "Y"=0.012237268012254776}, {"X"=17.34, "Y"=-0.035170220884613954}, {"X"=17.35, "Y"=-0.025811334900431738}, {"X"=17.36, "Y"=-0.02574689519367853}, {"X"=17.37, "Y"=0.03327897198554506}, {"X"=17.38, "Y"=-0.004400592958369716}, {"X"=17.39, "Y"=-0.007664359385141273}, {"X"=17.4, "Y"=0.0288089834941938}, {"X"=17.41, "Y"=0.014712500659707715}, {"X"=17.42, "Y"=-0.02539319722619913}, {"X"=17.43, "Y"=0.037378142377218385}, {"X"=17.44, "Y"=-0.04164575306335689}, {"X"=17.45, "Y"=0.012024154964659172}, {"X"=17.46, "Y"=0.00082290569938176}, {"X"=17.47, "Y"=0.039837434696515586}, {"X"=17.48, "Y"=0.046460502182404585}, {"X"=17.490000000000002, "Y"=0.02162736514558287}, {"X"=17.5, "Y"=0.011597343950906003}, {"X"=17.51, "Y"=-0.009311271507712956}, {"X"=17.52, "Y"=-0.005699218447667134}, {"X"=17.53, "Y"=-0.012073461599898229}, {"X"=17.54, "Y"=-0.009704620790551198}, {"X"=17.55, "Y"=-0.019035072694693133}, {"X"=17.56, "Y"=-0.004347344075287866}, {"X"=17.57, "Y"=0.01726792000345768}, {"X"=17.580000000000002, "Y"=0.0021163300590548713}, {"X"=17.59, "Y"=-0.03555884710917821}, {"X"=17.6, "Y"=0.011771277608873452}, {"X"=17.61, "Y"=-0.0010434939497805725}, {"X"=17.62, "Y"=0.003947595546438949}, {"X"=17.63, "Y"=-0.002878553350577455}, {"X"=17.64, "Y"=0.006100084105032709}, {"X"=17.65, "Y"=0.0022808048315499175}, {"X"=17.66, "Y"=-0.026016594245692526}, {"X"=17.67, "Y"=-0.02599403316293187}, {"X"=17.68, "Y"=-0.025161522071350872}, {"X"=17.69, "Y"=-0.019091355247974336}, {"X"=17.7, "Y"=-0.008819304806693181}, {"X"=17.71, "Y"=0.015406847526945868}, {"X"=17.72, "Y"=0.011093639502705347}, {"X"=17.73, "Y"=-0.012918017703402212}, {"X"=17.740000000000002, "Y"=0.009372331389010492}, {"X"=17.75, "Y"=0.0203289900777718}, {"X"=17.76, "Y"=-0.0031319580917262085}, {"X"=17.77, "Y"=-0.03161388631798681}, {"X"=17.78, "Y"=0.004242188918311331}, {"X"=17.79, "Y"=-0.0045099095343171455}, {"X"=17.8, "Y"=-0.005366418865078187}, {"X"=17.81, "Y"=0.005736081303599743}, {"X"=17.82, "Y"=0.0038247283992204366}, {"X"=17.830000000000002, "Y"=0.010540977497661072}, {"X"=17.84, "Y"=-0.02891630598480006}, {"X"=17.85, "Y"=0.04584203177167878}, {"X"=17.86, "Y"=0.042030007389700565}, {"X"=17.87, "Y"=0.006915122065451247}, {"X"=17.88, "Y"=0.003035581456369854}, {"X"=17.89, "Y"=-0.01627311423087431}, {"X"=17.9, "Y"=-0.0033046165701934183}, {"X"=17.91, "Y"=0.009561768187260459}, {"X"=17.92, "Y"=-0.012029753674451183}, {"X"=17.93, "Y"=-0.00839484809870479}, {"X"=17.94, "Y"=0.027375676550777085}, {"X"=17.95, "Y"=0.00642798332677266}, {"X"=17.96, "Y"=0.002716765142970264}, {"X"=17.97, "Y"=-0.03401716659628003}, {"X"=17.98, "Y"=0.029919698769656045}, {"X"=17.990000000000002, "Y"=0.004666755809839126}, {"X"=18.0, "Y"=-0.0007347427573465024}, {"X"=18.01, "Y"=-0.01903557410251286}, {"X"=18.02, "Y"=0.03824040318024898}, {"X"=18.03, "Y"=0.021453896727017745}, {"X"=18.04, "Y"=-0.00044907804686170386}, {"X"=18.05, "Y"=-0.024104505629034448}, {"X"=18.06, "Y"=0.006033774451020502}, {"X"=18.07, "Y"=0.013379229843387625}, {"X"=18.080000000000002, "Y"=0.01431586813805567}, {"X"=18.09, "Y"=-0.015272658855340362}, {"X"=18.1, "Y"=-0.0017100737071904977}, {"X"=18.11, "Y"=-0.03237458930361028}, {"X"=18.12, "Y"=0.03450487845505146}, {"X"=18.13, "Y"=-0.00736728453668979}, {"X"=18.14, "Y"=0.0417648290068835}, {"X"=18.150000000000002, "Y"=-0.010987546377480728}, {"X"=18.16, "Y"=-0.01402052289742454}, {"X"=18.17, "Y"=0.021030459784614642}, {"X"=18.18, "Y"=0.03199487299741259}, {"X"=18.19, "Y"=0.048357037008360866}, {"X"=18.2, "Y"=-0.01959763720156938}, {"X"=18.21, "Y"=0.023742201399197034}, {"X"=18.22, "Y"=-0.05891312303444679}, {"X"=18.23, "Y"=0.014410625380153329}, {"X"=18.240000000000002, "Y"=-0.026392960219290582}, {"X"=18.25, "Y"=0.0037872495730903594}, {"X"=18.26, "Y"=0.005238817489214101}, {"X"=18.27, "Y"=-0.024079173258501493}, {"X"=18.28, "Y"=0.011764902576723635}, {"X"=18.29, "Y"=0.024700173667642728}, {"X"=18.3, "Y"=0.018037298253293976}, {"X"=18.31, "Y"=-0.00612472617200936}, {"X"=18.32, "Y"=-0.003843794743441033}, {"X"=18.330000000000002, "Y"=-0.04153982037253531}, {"X"=18.34, "Y"=0.004053225733190619}, {"X"=18.35, "Y"=0.023451828340499997}, {"X"=18.36, "Y"=-0.004725317978281292}, {"X"=18.37, "Y"=-0.01434278467575656}, {"X"=18.38, "Y"=-0.005942067927948687}, {"X"=18.39, "Y"=0.031244930859985164}, {"X"=18.400000000000002, "Y"=0.002191425166889199}, {"X"=18.41, "Y"=-0.0022272769234243585}, {"X"=18.42, "Y"=0.021634328165136746}, {"X"=18.43, "Y"=-0.007144302291749539}, {"X"=18.44, "Y"=-0.005436233846580882}, {"X"=18.45, "Y"=0.012161483252513662}, {"X"=18.46, "Y"=-0.027404338988751064}, {"X"=18.47, "Y"=0.0381525566406267}, {"X"=18.48, "Y"=0.01663224193671437}, {"X"=18.490000000000002, "Y"=0.059465045624041535}, {"X"=18.5, "Y"=-0.010203834698620299}, {"X"=18.51, "Y"=-0.03722469423236966}, {"X"=18.52, "Y"=-0.003176728411367004}, {"X"=18.53, "Y"=0.01918310159658008}, {"X"=18.54, "Y"=0.008400991045101351}, {"X"=18.55, "Y"=-0.00817287089029598}, {"X"=18.56, "Y"=-0.028113571280905303}, {"X"=18.57, "Y"=0.021081038547283024}, {"X"=18.580000000000002, "Y"=-0.018201448965352265}, {"X"=18.59, "Y"=0.0415072952381082}, {"X"=18.6, "Y"=-0.002755075670612776}, {"X"=18.61, "Y"=-0.0021980363719047878}, {"X"=18.62, "Y"=0.022469416310463043}, {"X"=18.63, "Y"=0.02944687698226081}, {"X"=18.64, "Y"=-0.0317674025913958}, {"X"=18.650000000000002, "Y"=-0.012379104211822967}, {"X"=18.66, "Y"=0.047038079693039886}, {"X"=18.67, "Y"=-0.026060608358528182}, {"X"=18.68, "Y"=-0.0016169472272392882}, {"X"=18.69, "Y"=0.020624893498608382}, {"X"=18.7, "Y"=-0.01760757425391402}, {"X"=18.71, "Y"=-0.011737882457055081}, {"X"=18.72, "Y"=0.017020639746995476}, {"X"=18.73, "Y"=0.010161770628607712}, {"X"=18.740000000000002, "Y"=0.014909266699720227}, {"X"=18.75, "Y"=0.041969275977600876}, {"X"=18.76, "Y"=0.008965872869607271}, {"X"=18.77, "Y"=0.030706345085279255}, {"X"=18.78, "Y"=-0.0221404178664905}, {"X"=18.79, "Y"=-0.021349971298256915}, {"X"=18.8, "Y"=0.02623083742387345}, {"X"=18.81, "Y"=-0.03884236746874354}, {"X"=18.82, "Y"=0.02595777594871552}, {"X"=18.830000000000002, "Y"=0.010750642833746264}, {"X"=18.84, "Y"=0.006690956839875982}, {"X"=18.85, "Y"=-0.04020963004623038}, {"X"=18.86, "Y"=-0.007745041508812259}, {"X"=18.87, "Y"=-0.018890836982704107}, {"X"=18.88, "Y"=-0.009742441277288953}, {"X"=18.89, "Y"=-0.023604414488414334}, {"X"=18.900000000000002, "Y"=0.015837059176956526}, {"X"=18.91, "Y"=0.008546308462339777}, {"X"=18.92, "Y"=-0.0031550698198050207}, {"X"=18.93, "Y"=0.03626511276618092}, {"X"=18.94, "Y"=0.04285658837442547}, {"X"=18.95, "Y"=-0.04539724313153321}, {"X"=18.96, "Y"=-0.019692493680294253}, {"X"=18.97, "Y"=-0.00876973816460923}, {"X"=18.98, "Y"=0.01114952894766247}, {"X"=18.990000000000002, "Y"=0.011454398588120232}, {"X"=19.0, "Y"=-0.02496549181923227}]
  in  "Tab Control":enum32{"Frequency", "Digitizer", "Error"}(tab)
  in  "Power dBm":dbl=10.0
  in  "Frequency diff MHz":dbl=50.0
  in  "End GHz":dbl=19.0
  in  "Step GHz":dbl=0.01
  in  "Start Frequency GHz":dbl=1.0
  in  "Cold Start LO":bool
  in  "M nChannel":i32=1
  in  "Ref nChannel":i32=2
  in  "Enable Ref Channel":bool=TRUE
  in  "DAQ parameter":T1={"cycles"=1, "points"=2000, "triggerMode"=0, "triggerDelay"=0} {"triggerMode" items=["Auto", "VI/HVI", "External", "Analog"]; "cycles" min=0}
  in  "Channel parameter":T2={"fullscale"=0.125, "impedance"=1, "coupling"=0} {"coupling" items=["DC", "AC"]; "impedance" items=["High Z", "50 Ohms"]; "fullscale" items=["0.0625"=0.0625, "0.125"=0.125, "0.25"=0.25, "0.5"=0.5, "1"=1.0, "2"=2.0, "4"=4.0]}
  out "errorOut":errorcluster
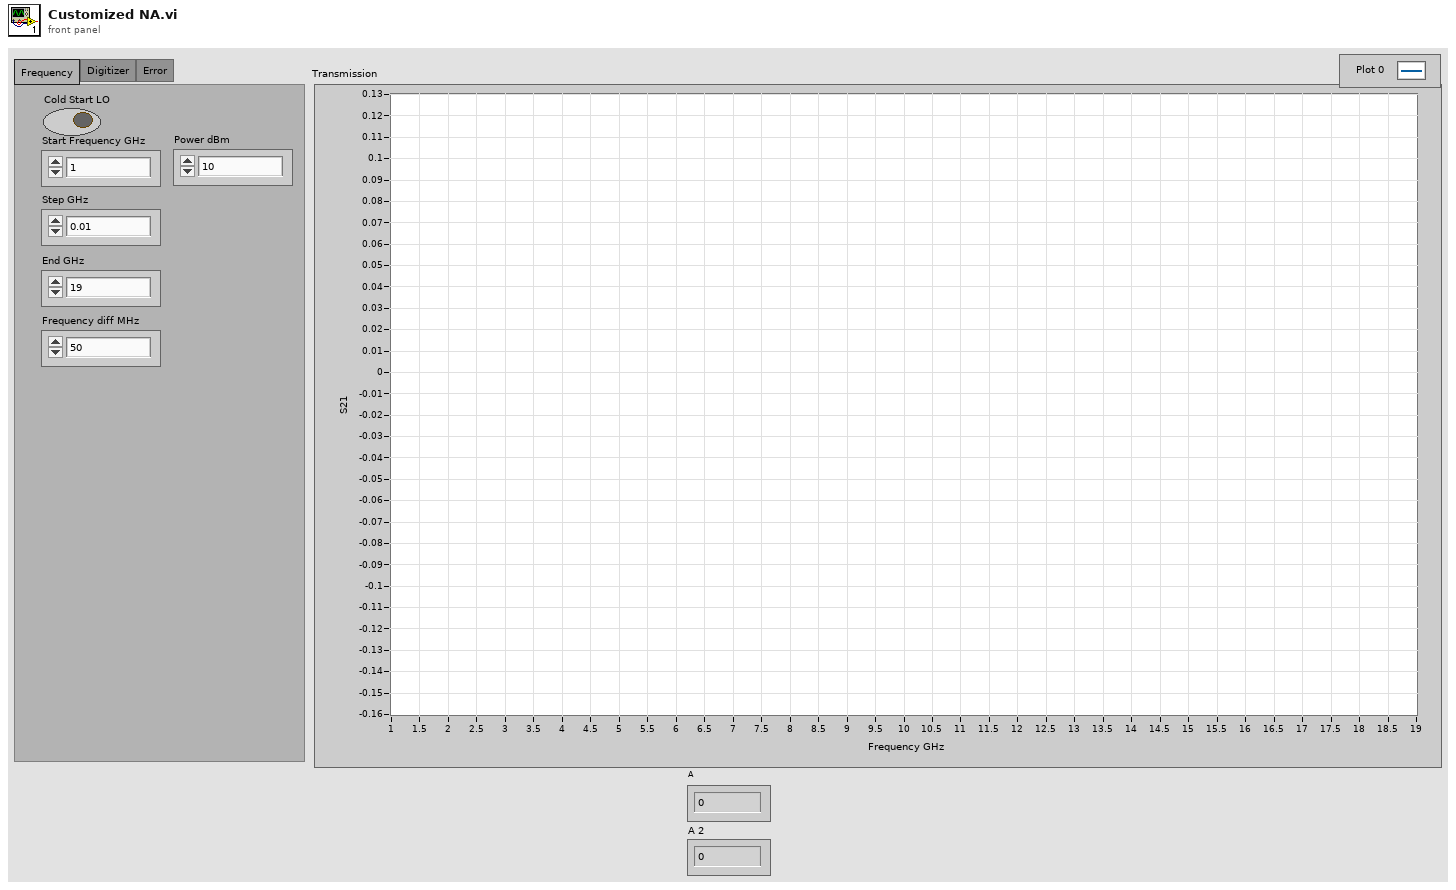
[diagram p1: front panel]
types:
  T1 = cluster{"cycles":i32, "points":i32, "triggerMode":i32, "triggerDelay":i32}
  T2 = cluster{"fullscale":dbl, "impedance":i32, "coupling":i32}
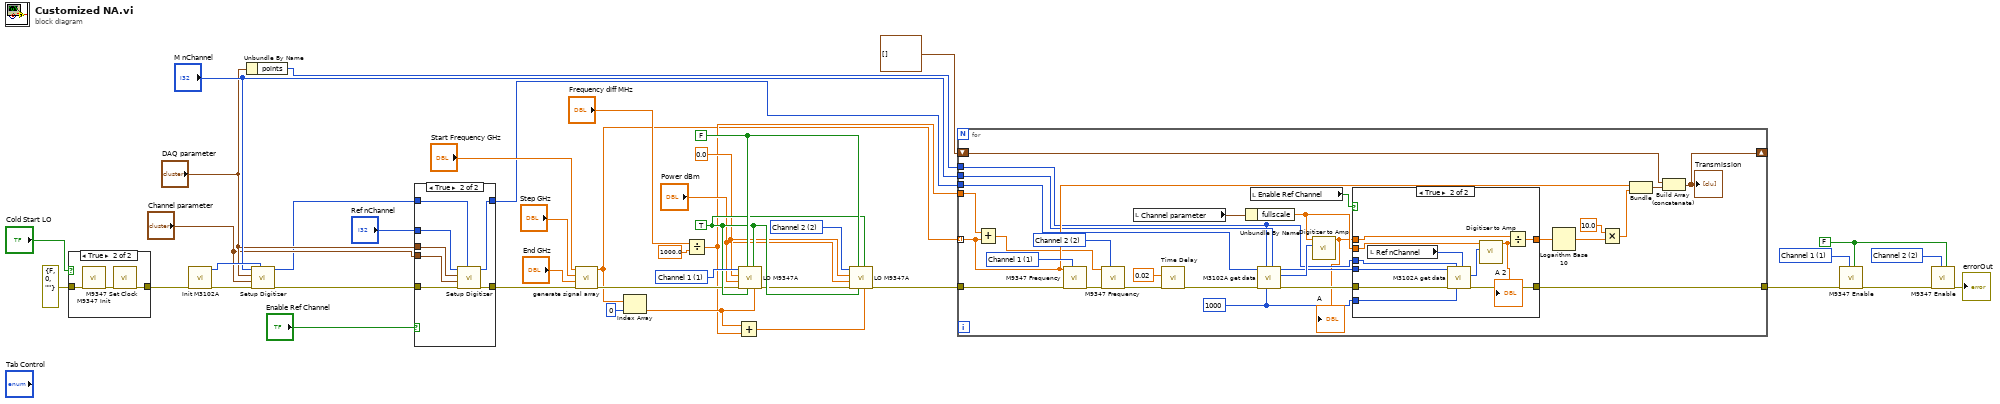
[diagram p0: block diagram]
diagram:
  w3 = u16 2 items=["Channel 2"=2, "Channel 1"=1] ("Chan")
  w4 = u16 1 items=["Channel 2"=2, "Channel 1"=1] ("Chan")
  w5 = FALSE ("Enable")
  w32 = 0.0 ("Phase degree")
  w35 = u16 2 items=["Channel 2"=2, "Channel 1"=1] ("Chan")
  w36 = u16 1 items=["Channel 2"=2, "Channel 1"=1] ("Chan")
  w33 = TRUE ("Exec")
  w34 = FALSE ("Init")
  n1 = case shown="True" "Cold Start LO" {
    tunnel: errorcluster {"status"=FALSE, "code"=0, "source"=""} ("error in") -> [w42 w45]
    tunnel: [w42 w43] -> w21
    frame False {
    }
    frame True {
      n2 = call "M9347 Init.vi"("error in (no error)"=w45) -> ("error out"=w44:errorcluster)  [unwired: 10 in]
      n3 = call "M9347 Set Clock.vi"("error in (no error)"=w44) -> ("error out"=w43:errorcluster)  [unwired: 10 in]
    }
  }
  n4 = call "Init M3102A.vi"("errorIn"=w21) -> ("errorOut"=w16:errorcluster, "moduleID"=w17:i32)  [unwired: 9 in]
  n5 = Unbundle By Name("DAQ parameter") -> ("points"=w1:i32)
  n6 = call "Setup Digitizer.vi"("moduleID"=w17, "error in (no error)"=w16, "Channel M"="Channel parameter", "DAQ M"="DAQ parameter", "nChannel"="M nChannel") -> ("error out"=w11:errorcluster, "Digitizer ID"=w9:i32)  [unwired: 5 in]
  n7 = case shown="True" "Enable Ref Channel" {
    tunnel: "Ref nChannel" -> [_ w54]
    tunnel: "DAQ parameter" -> [_ w53]
    tunnel: "Channel parameter" -> [_ w52]
    tunnel: w11 -> [w47 w51]
    tunnel: [w47 w50] -> w10
    tunnel: w9 -> [w46 w49]
    tunnel: [w46 w48] -> w8
    frame False {
    }
    frame True {
      n8 = call "Setup Digitizer.vi"("moduleID"=w49, "error in (no error)"=w51, "Channel M"=w52, "DAQ M"=w53, "nChannel"=w54) -> ("error out"=w50:errorcluster, "Digitizer ID"=w48:i32)  [unwired: 5 in]
    }
  }
  n9 = call "generate signal array.vi"("error in"=w10, "End"="End GHz", "Step"="Step GHz", "Start"="Start Frequency GHz") -> ("error out"=w24:errorcluster, "Output"=w20:dbl[])  [unwired: 6 in]
  n10 = Index Array(array=w20, index=0) -> (element=w29:dbl)
  n11 = Divide(x="Frequency diff MHz", y=1000.0) -> (x/y=w22:dbl)
  n12 = Add(x=w29, y=w22) -> (x+y=w26:dbl)
  n13 = call "LO M9347A.vi"("Frequency GHz"=w29, "Exec"=w33, "Enable"=w33, "Init"=w34, "error in (no error)"=w24, "Power dBm"="Power dBm", "Phase degree"=w32, "Chan"=w36) -> ("error out"=w25:errorcluster)  [unwired: 3 in]
  n14 = call "LO M9347A.vi"("Frequency GHz"=w26, "Exec"=w33, "Enable"=w33, "Init"=w34, "error in (no error)"=w25, "Power dBm"="Power dBm", "Phase degree"=w32, "Chan"=w35) -> ("error out"=w23:errorcluster)  [unwired: 3 in]
  n15 = for {
    tunnel: w23 -> [w83]
    tunnel: w20 -> [w73] mode=indexing
    tunnel: w22 -> [w72]
    tunnel: w8 -> [w76]
    tunnel: w1 -> [w64]
    tunnel: "M nChannel" -> [w66]
    shift-right: [w69] -> _
    shift-left: cluster{"Numeric":dbl, "A":dbl}[] [] -> [w68]
    tunnel: [w61] -> w7
    w65 = 1000 ("TimeOut")
    w80 = u16 2 items=["Channel 2"=2, "Channel 1"=1] ("Chan")
    w82 = u16 1 items=["Channel 2"=2, "Channel 1"=1] ("Chan")
    n16 = Add(x=w72, y=w73) -> (x+y=w71:dbl)
    n17 = call "M9347 Frequency.vi"("Chan"=w82, "error in (no error)"=w83, "Frequency GHz"=w73) -> ("error out"=w81:errorcluster)  [unwired: 8 in]
    n18 = call "M9347 Frequency.vi"("Chan"=w80, "error in (no error)"=w81, "Frequency GHz"=w71) -> ("error out"=w79:errorcluster)  [unwired: 8 in]
    n19 = local read "Channel parameter"() -> (w74:T2)
    n20 = call "Time Delay"("error in (no error)"=w79, "Delay Time (s)"=0.02) -> ("error out"=w77:errorcluster)  [unwired: 9 in]
    n21 = Unbundle By Name(w74) -> ("fullscale"=w60:dbl)
    n22 = local read "Enable Ref Channel"() -> (w67:bool)
    n23 = call "M3102A get data.vi"("channel number"=w66, "TimeOut"=w65, "DAQpoints"=w64, "errorIn"=w77, "moduleID"=w76) -> ("errorOut"=w63:errorcluster, "DAQdata"=w75:i16[], "moduleIDout"=w62:i32)  [unwired: 4 in]
    n24 = call "Digitizer to Amp.vi"("DAQdata"=w75, "fullscale"=w60) -> ("A"=w55:dbl)  [unwired: 9 in]
    "A" <- w55
    n25 = case shown="True" w67 {
      tunnel: w65 -> [_ w96]
      tunnel: w64 -> [_ w95]
      tunnel: w63 -> [w84 w94]
      tunnel: w62 -> [_ w93]
      tunnel: [w84 w92] -> w61
      tunnel: w60 -> [_ w90]
      tunnel: [w85 w88] -> w59
      tunnel: w55 -> [w85 w89]
      frame False {
      }
      frame True {
        n26 = local read "Ref nChannel"() -> (w87:i32)
        n27 = call "M3102A get data.vi"("channel number"=w87, "TimeOut"=w96, "DAQpoints"=w95, "errorIn"=w94, "moduleID"=w93) -> ("errorOut"=w92:errorcluster, "DAQdata"=w91:i16[])  [unwired: 4 in, 1 out]
        n28 = call "Digitizer to Amp.vi"("DAQdata"=w91, "fullscale"=w90) -> ("A"=w86:dbl)  [unwired: 9 in]
        "A 2" <- w86
        n29 = Divide(x=w89, y=w86) -> (x/y=w88:dbl)
      }
    }
    n30 = Logarithm Base 10(1:w59) -> (0:w58:dbl)
    n31 = Multiply(x=10.0, y=w58) -> (x*y=w56:dbl)
    n32 = Bundle("Numeric"=w73, w56) -> (w70:cluster{"Numeric":dbl, dbl})  [unwired: 1 in]
    n33 = Build Array (concatenate)(w68, w70) -> (w69:cluster{"Numeric":dbl, "A":dbl}[])
    "Transmission" <- w69
  }
  n34 = call "M9347 Enable.vi"("Enable"=w5, "Chan"=w4, "error in (no error)"=w7) -> ("error out"=w6:errorcluster)  [unwired: 8 in]
  n35 = call "M9347 Enable.vi"("Enable"=w5, "Chan"=w3, "error in (no error)"=w6) -> ("error out"=→"errorOut":errorcluster)  [unwired: 8 in]
